vi "STED Control V1.vi"() -> ()   [LabVIEW 2014]
uses:
  FPGA-7842R-Reference.ctl
  Scan Parameters.ctl
  Manual Controls V2.ctl
  <vilib>/Utility/miscctls.llb/LVRectTypeDef.ctl
  <vilib>/Utility/miscctls.llb/LVPositionTypeDef.ctl
  Laser Controls.ctl
  Type Defs/Image Acquisition Parameters.ctl
  Detectors.ctl
panel:
  in  "Move XY Stage":bool
  in  "Autoscale Z":bool
  in  "Reset Zoom":bool
  in  "Zoom Out":bool
  in  "Zoom In":bool
  in  "Pan":bool
  in  "Remove Display":bool
  in  "Add Display":bool
  in  "Colormap 2":u16(ring) items=["Fire", "Gray", "Red", "Green", "Blue", "Cyan", "Magenta", "Yellow", "Red-White", "Green-White", "Blue-White", "Glow"]
  in  "Merge Tool":bool
  in  "Smooth Tool":bool
  out "Channel 6":sgl[][](graph)
  out "Channel 5":sgl[][](graph)
  out "Channel 4":sgl[][](graph)
  out "Channel 3":sgl[][](graph)
  out "Channel 2":sgl[][](graph)
  in  "Dual Screens":bool=TRUE
  in  "Detectors":T1
  in  "Laser Controls":T2 {"590 Power (V)" scale=0.0..3.0; "STED Power (V)" scale=0.0..5.0}
  in  "Save File Path":path
  in  "Capture":bool
  in  "show cursor":bool
  in  "Set Mode Offset":bool
  in  "Manual Controls":T3={"Galvo 1 Position (I16)"=-280, "Galvo 2 Position (I16)"=0, "X Axis Voltage (I16)"=16384, "Y Axis Voltage (I16)"=16384, "Z Axis Voltage (I16)"=16384, "Res Mirror Amp (I16)"=0, "Res Mirror Mute"=FALSE}
  in  "Unused Axis Voltage":i16=16300
  out "Channel 1":sgl[][](graph)
  in  "Image Acquisition Parameters":T4={"Scan Type"=enum."Sample Scanning", "Scan Mode"=enum."XY", "Fast Axis Frequency (Hz)"=100.0, "Image Format"=128, "Line Accumulations"=1, "Frames Per Capture"=1, "Frames Accumulations"=1, "Image Dimension (um)"=[], "Number of Z Steps"=1, "Z Steps Size (um)"=1.0, "Pixel Size (nm)"=[]} {"Z Steps Size (um)" min=0.0; "Number of Z Steps" min=1; "Frames Accumulations" min=1; "Frames Per Capture" min=1; "Line Accumulations" min=1; "Image Format" items=["64 x 64"=64, "128 x 128"=128, "256 x 256"=256, "512 x 512"=512, "1024 x 1024"=1024, "2048 x 2048"=2048]}
  in  "Live":bool
  in  "Exit":bool
  # "XY"
  # "Z"
  # "Length"
  # "Height"
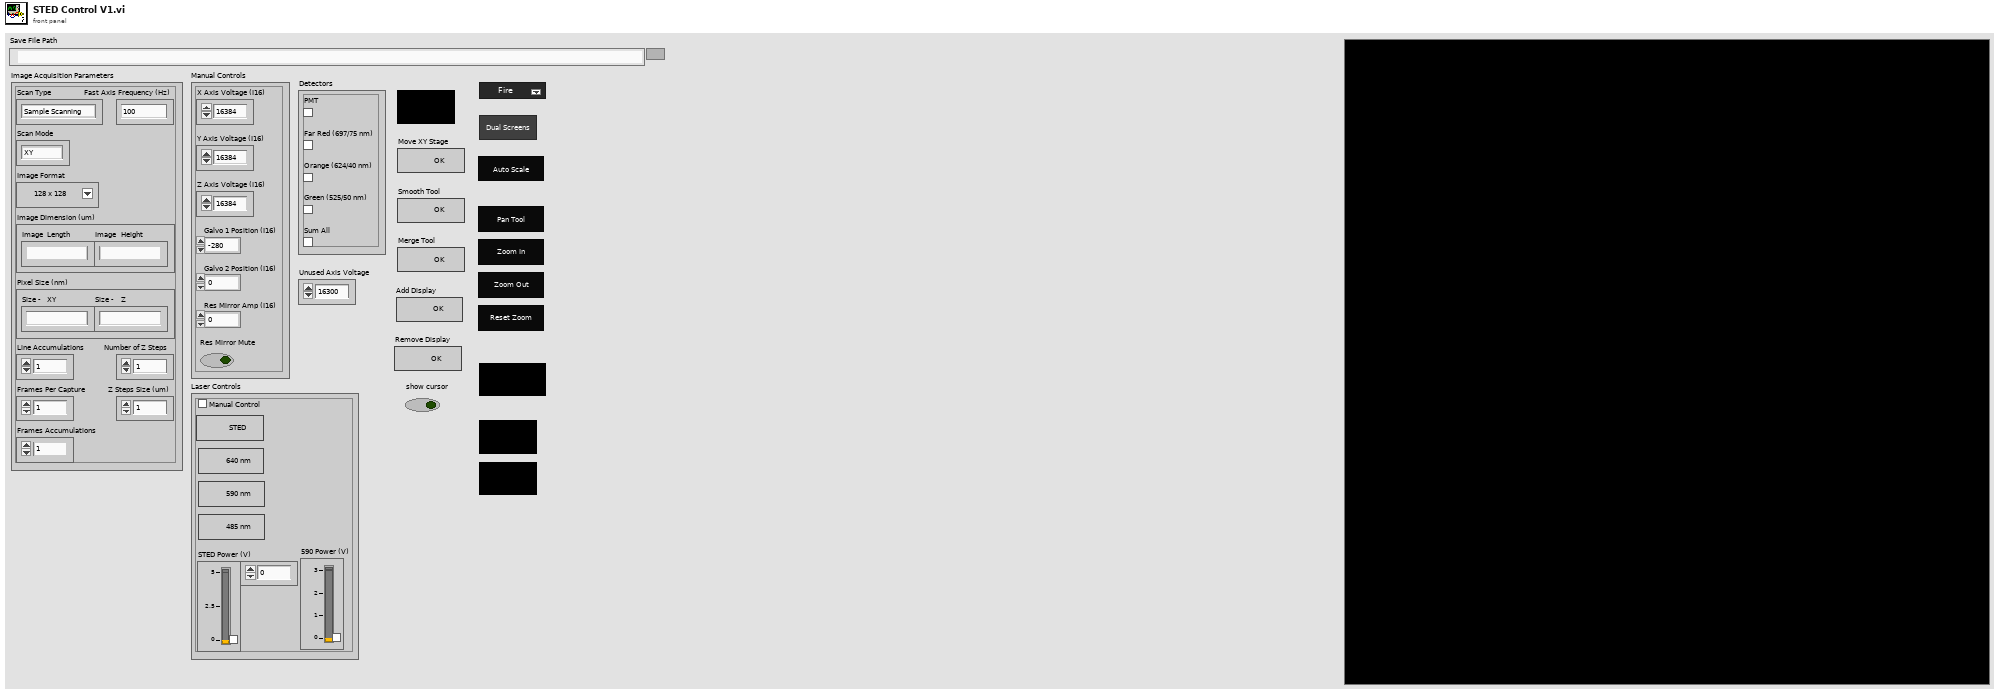
[diagram p1: front panel]
types:
  T1 = typedef "Detectors.ctl" = cluster{"PMT":bool, "Far Red (697/75 nm)":bool, "Orange (624/40 nm)":bool, "Green (525/50 nm)":bool, "Sum All":bool}
  T2 = typedef "Laser Controls.ctl" = cluster{"STED Power (V)":dbl, "590 Power (V)":dbl, "STED":bool, "640 nm":bool, "590 nm":bool, "485 nm":bool, "Manual Control":bool}
  T3 = typedef "Manual Controls V2.ctl" = cluster{"Galvo 1 Position (I16)":i16, "Galvo 2 Position (I16)":i16, "X Axis Voltage (I16)":i16, "Y Axis Voltage (I16)":i16, "Z Axis Voltage (I16)":i16, "Res Mirror Amp (I16)":i16, "Res Mirror Mute":bool}
  T4 = typedef "Image Acquisition Parameters.ctl" = cluster{"Scan Type":enum16{"Sample Scanning", "Beam Scanning"}, "Scan Mode":enum16{"XY", "XZ", "YZ", "XYZ"}, "Fast Axis Frequency (Hz)":dbl, "Image Format":u16, "Line Accumulations":u16, "Frames Per Capture":u16, "Frames Accumulations":u16, "Image Dimension (um)":dbl[], "Number of Z Steps":u8, "Z Steps Size (um)":dbl, "Pixel Size (nm)":dbl[]}
  T5 = typedef "Scan Parameters.ctl" = cluster{"Fast_Ax_Amp_V":dbl, "Fast_Ax_Off_V":dbl, "Slow_Ax_Amp_V":dbl, "Slow_Ax_Off_V ":dbl, "Slow_Ax_Max_V_VperS":dbl, "Slow_Ax1_Del25ns":i32, "Slow_Ax2_Del25ns":i32, "Stage_X_Off_V":dbl, "Stage_Y_Off_V":dbl, "Stage_Z_Off_V":dbl, "Galvo1_Off_V":dbl, "Galvo2_Off_V":dbl, "Last_Scan_Mode":enum16{"XY", "XZ", "YZ", "XYZ"}, "Current_Scan_Mode":enum16{"XY", "XZ", "YZ", "XYZ"}, "Fly_Back_Lines":u16, "Linear_Ramp_End":u32, "Z_Step_I16":i16, "Z_Start_I16":i16, "Laser_States _U32":u32, "590_Voltage_I16":i16, "775_AOM_Volt_I16":i16, "Blanking OFF":bool, "Unused_Axis_I16":i16}
  T6 = typedef "FPGA-7842R-Reference.ctl" = enum16{"Stage Control", "Laser Control", "Unused Axis I16", "Exit", "Set Res Mirror", "Set Galvo", "Default", "Close FPGA", "Stop Waveforms", "Start Waveforms", "Initialize"}
  T7 = typedef "LVPositionTypeDef.ctl" = cluster{"Left":i32, "Top":i32}
  T8 = typedef "LVRectTypeDef.ctl" = cluster{"Left":i16, "Top":i16, "Right":i16, "Bottom":i16}
  T9 = enum32{"Invalid", "Standard", "Closed", "Hidden", "Minimized", "Maximized"}
  T10 = typedef "LVRangeTypeDef.ctl" = cluster{"Minimum":dbl, "Maximum":dbl, "Increment":dbl, "Minor Increment":dbl, "Start":dbl}
  T11 = cluster{"Galvo 1 Position (I16)":bool, "Galvo 2 Position (I16)":bool, "X Axis Voltage (I16)":bool, "Y Axis Voltage (I16)":bool, "Z Axis Voltage (I16)":bool, "Res Mirror Amp (I16)":bool, "Res Mirror Mute":bool}
  T12 = typedef "LVAllMonitorsDisplayTypeDef.ctl" = cluster{"Bounds":cluster{"Left":i16, "Top":i16, "Right":i16, "Bottom":i16}, "Depth":i16}[]
  T13 = cluster{"Bounds":cluster{"Left":i16, "Top":i16, "Right":i16, "Bottom":i16}, "Depth":i16}
  T14 = typedef "Scanning Conversions.ctl" = cluster{"Stage X Axis (Volts/um)":dbl, "Stage Y Axis (Volts/um)":dbl, "Stage Z Axis (Volts/um)":dbl}
  T15 = typedef "IMAQ Image.ctl" = refnum<image>
  T16 = typedef "Waveform Data.ctl" = cluster{"Waveform Scan Parameters":cluster{"Scanning Mode":u8, "Fast Axis WF Length (Elements)":i32, "Fast Axis Sample Period (Ticks)":u32, "Slow Axis 1 WF Length (Elements)":i32, "Slow Axis 1 Sample Period (Ticks)":u32, "Slow Axis 1 Delay (25 ns) Steps":i32, "Slow Axis 2 WFLength (Elements)":i32, "Slow Axis 2 Sample Period (Ticks)":u32, "Slow Axis 2 Delay (25 ns) Steps":i32}, "Fast Axis Waveform":dbl[], "Slow Axis 1 Waveform":dbl[], "Slow Axis 2 Waveform":dbl[]}
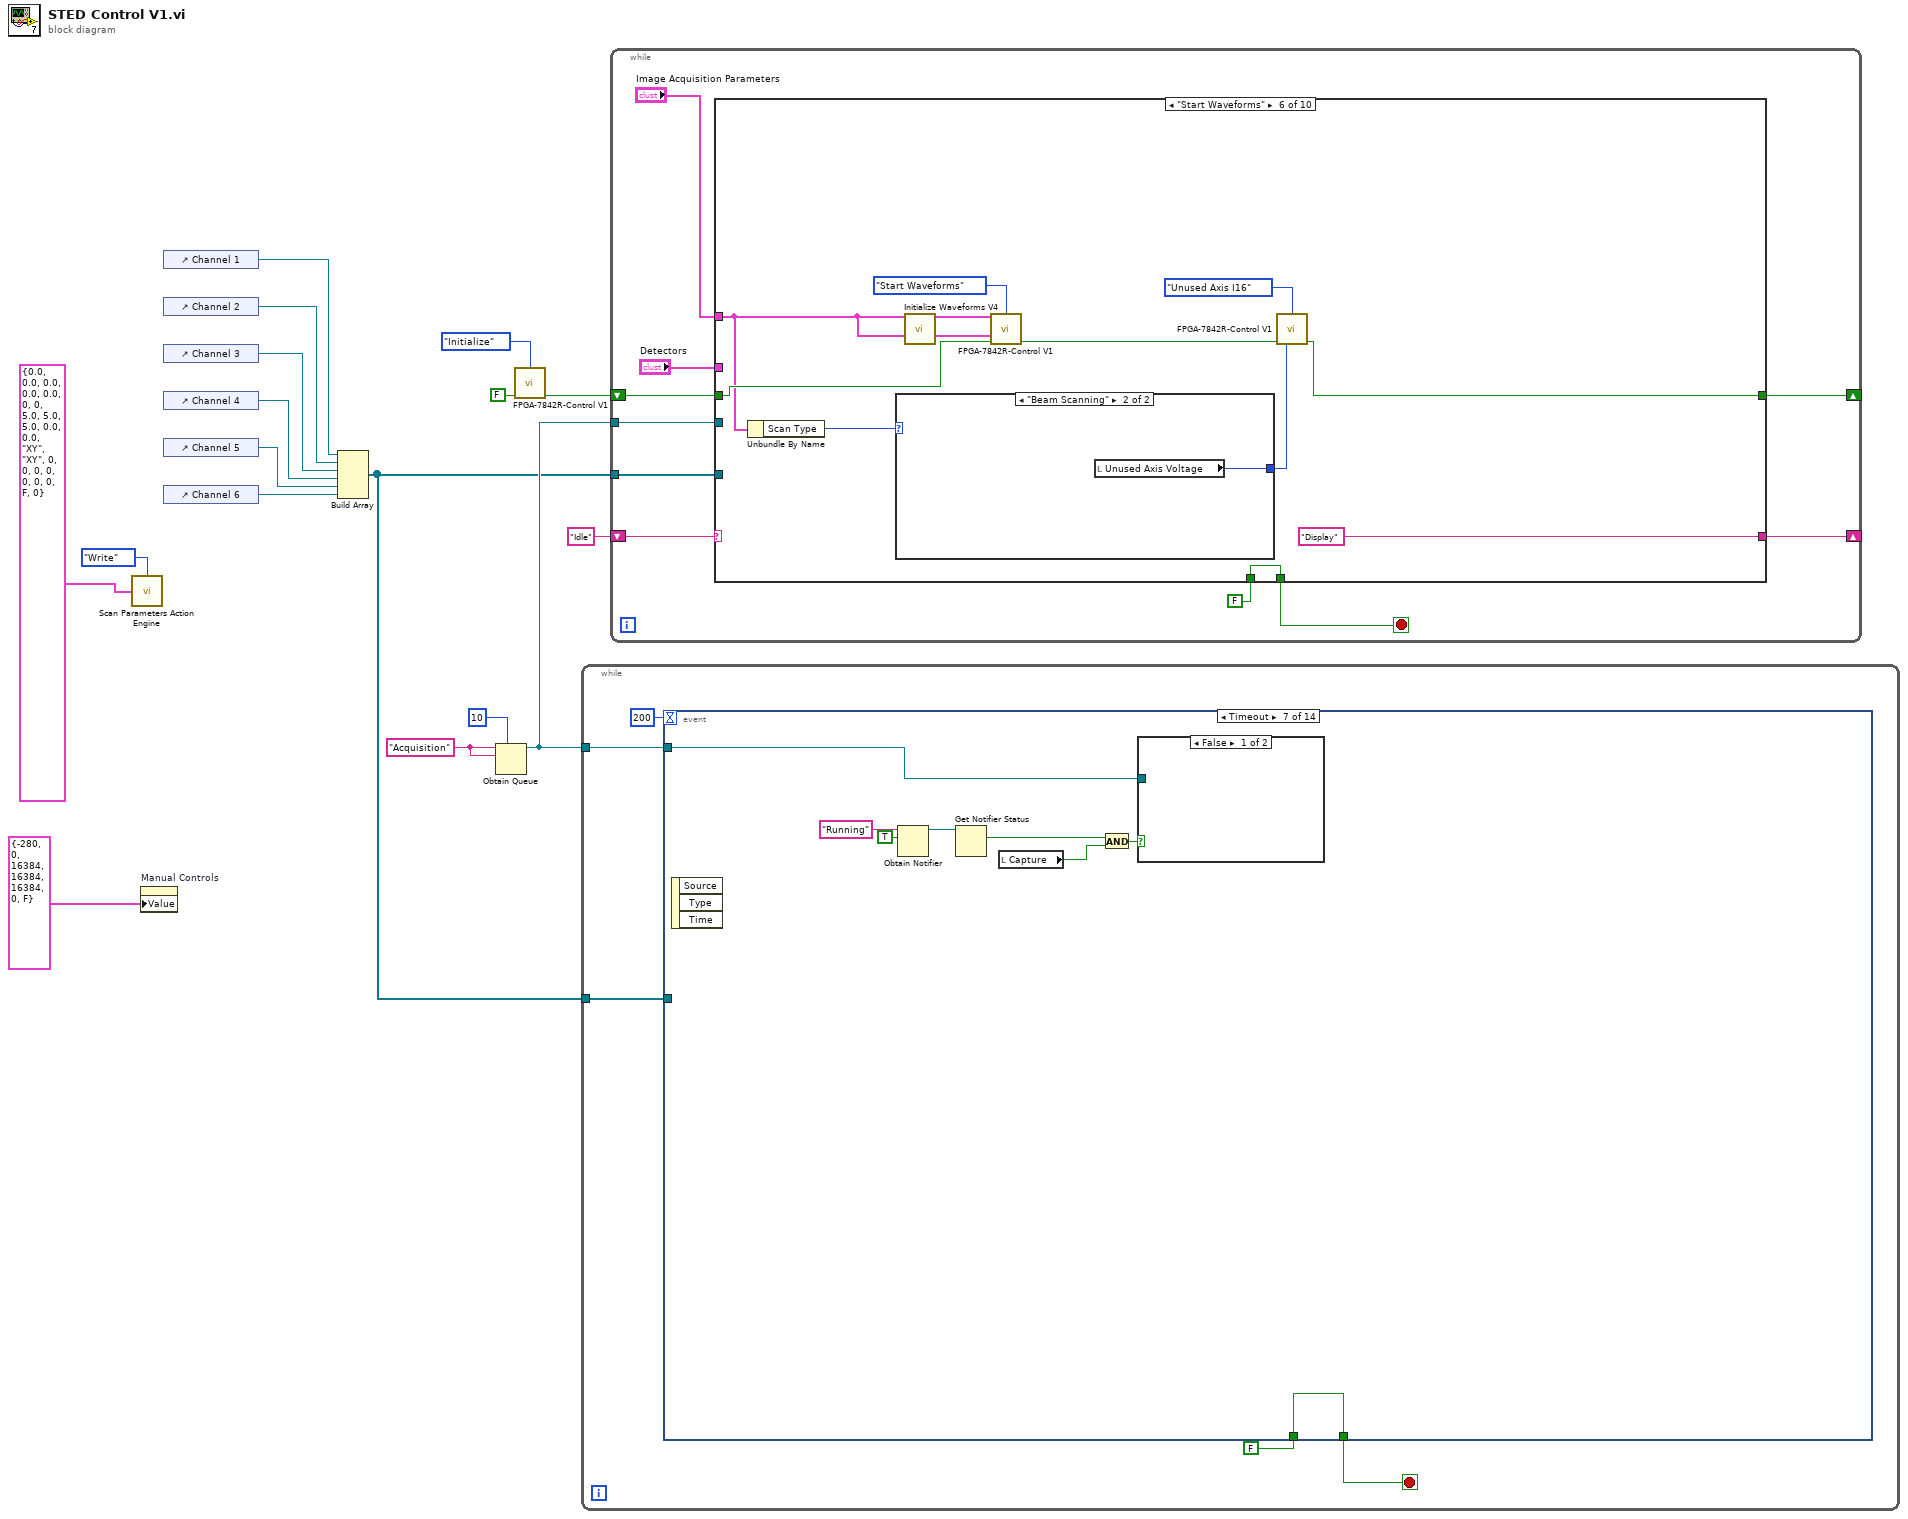
[diagram p0: block diagram]
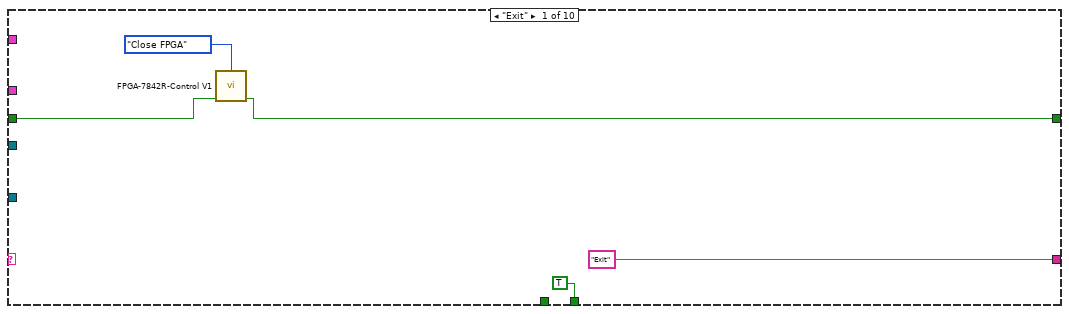
[diagram p2: hidden frame]
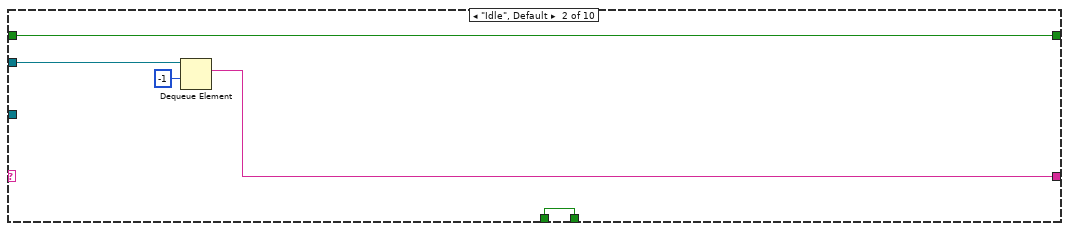
[diagram p3: hidden frame]
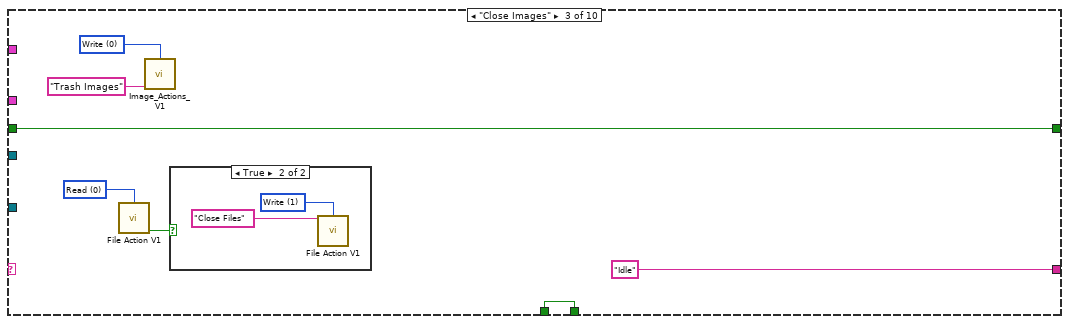
[diagram p4: hidden frame]
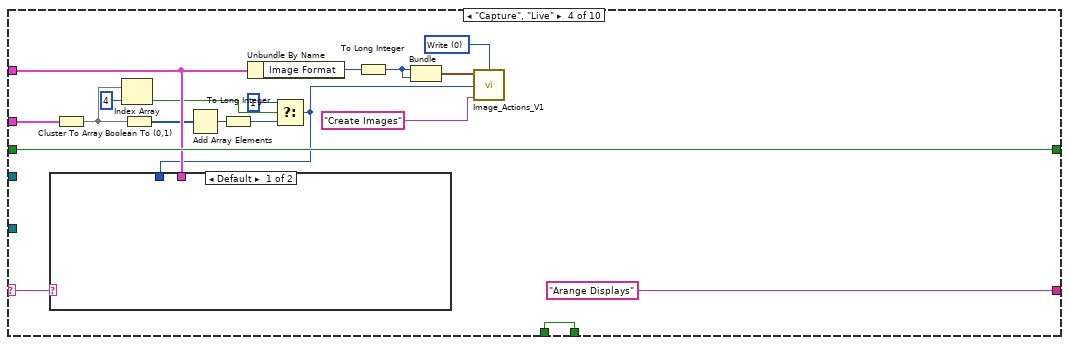
[diagram p6: hidden frame]
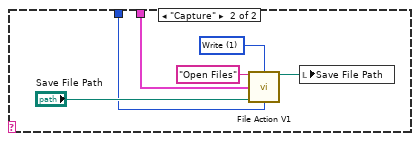
[diagram p7: hidden frame]
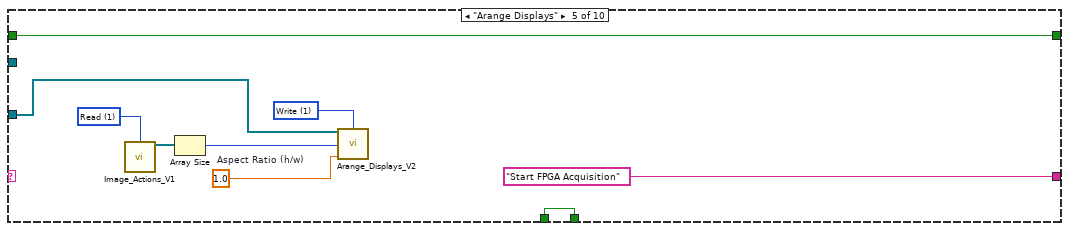
[diagram p8: hidden frame]
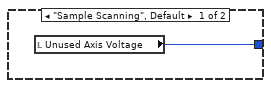
[diagram p9: hidden frame]
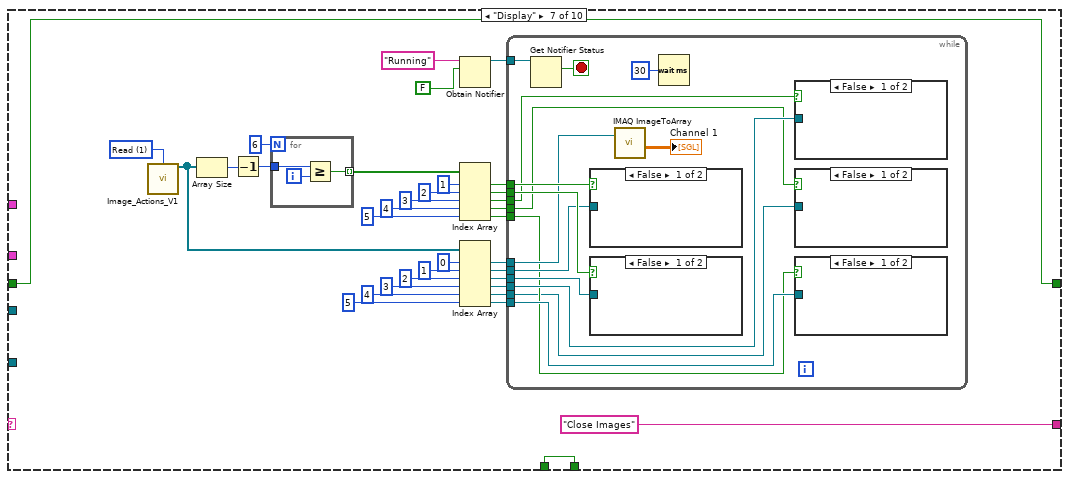
[diagram p10: hidden frame]
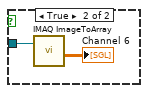
[diagram p11: hidden frame]
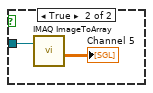
[diagram p12: hidden frame]
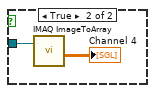
[diagram p13: hidden frame]
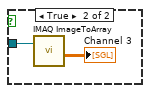
[diagram p14: hidden frame]
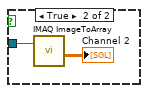
[diagram p15: hidden frame]
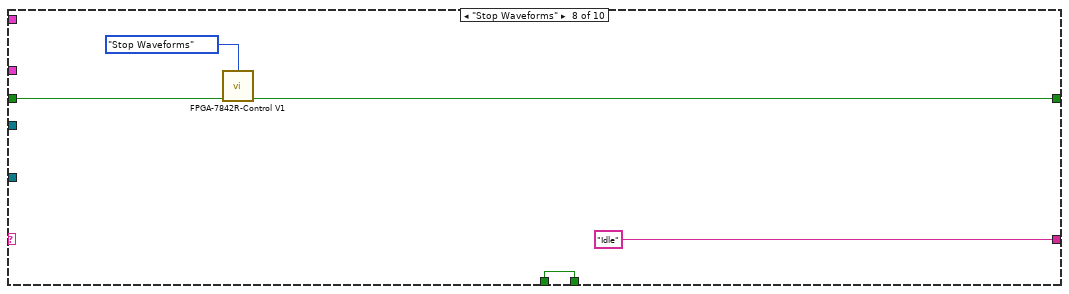
[diagram p16: hidden frame]
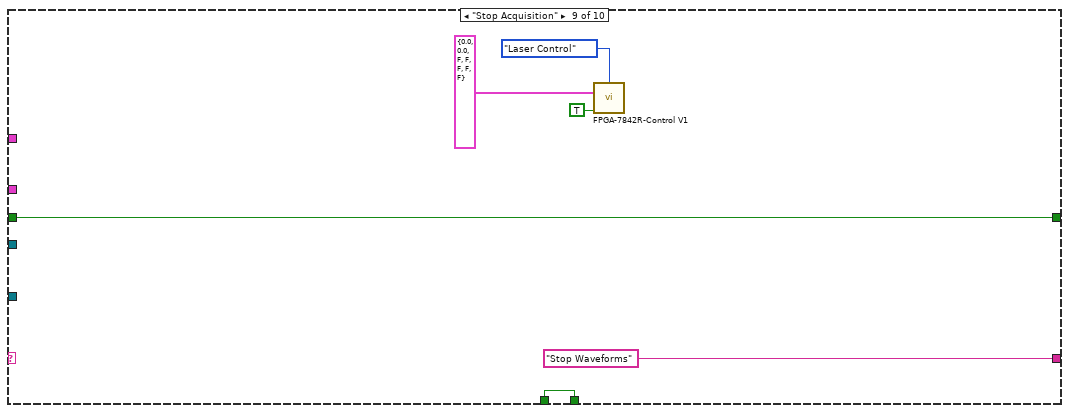
[diagram p17: hidden frame]
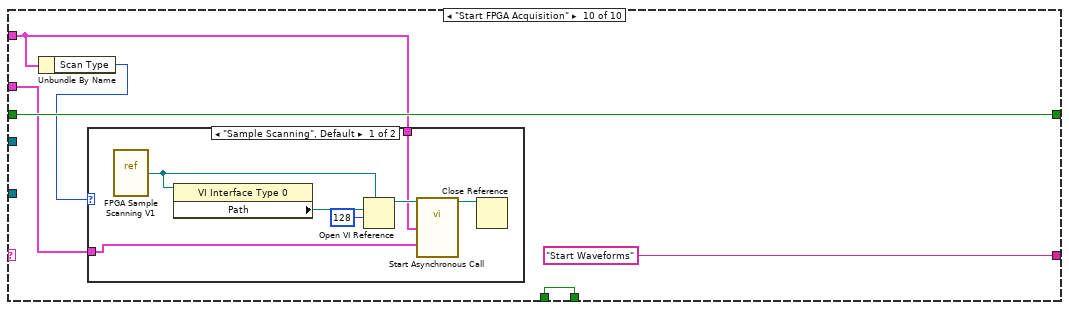
[diagram p18: hidden frame]
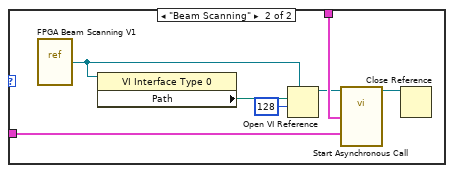
[diagram p19: hidden frame]
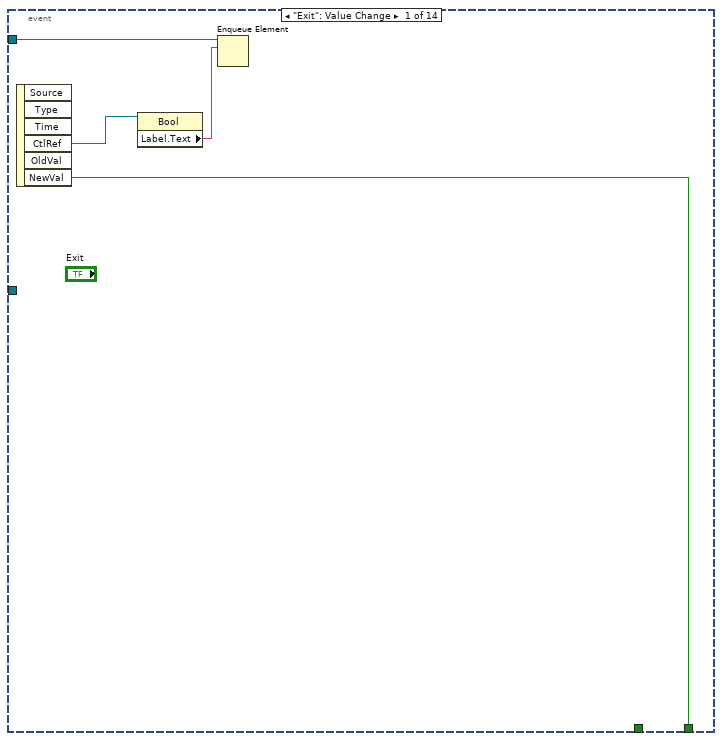
[diagram p20: hidden frame]
diagram:
  w16 = "Acquisition" ("name (unnamed)")
  n1 = call "Scan Parameters Action Engine.vi"("Action"=enum16{"Read", "Write"}."Write", "Scan Parameters IN"=T5 {"Fast_Ax_Amp_V"=0.0, "Fast_Ax_Off_V"=0.0, "Slow_Ax_Amp_V"=0.0, "Slow_Ax_Off_V "=0.0, "Slow_Ax_Max_V_VperS"=0.0, "Slow_Ax1_Del25ns"=0, "Slow_Ax2_Del25ns"=0, "Stage_X_Off_V"=5.0, "Stage_Y_Off_V"=5.0, "Stage_Z_Off_V"=5.0, "Galvo1_Off_V"=0.0, "Galvo2_Off_V"=0.0, "Last_Scan_Mode"=enum."XY", "Current_Scan_Mode"=enum."XY", "Fly_Back_Lines"=0, "Linear_Ramp_End"=0, "Z_Step_I16"=0, "Z_Start_I16"=0, "Laser_States _U32"=0, "590_Voltage_I16"=0, "775_AOM_Volt_I16"=0, "Blanking OFF"=FALSE, "Unused_Axis_I16"=0}) -> ()  [unwired: 13 in, 1 out]
  n2 = property on="Manual Controls" class="Clust (strict)"("Value"=T3 {"Galvo 1 Position (I16)"=-280, "Galvo 2 Position (I16)"=0, "X Axis Voltage (I16)"=16384, "Y Axis Voltage (I16)"=16384, "Z Axis Voltage (I16)"=16384, "Res Mirror Amp (I16)"=0, "Res Mirror Mute"=FALSE} ("Manual Controls")) -> ()  [unwired: 2 in, 2 out]
  n3 = control-ref of="Channel 1"() -> (w8:refnum<vi>)
  n4 = control-ref of="Channel 2"() -> (w7:refnum<vi>)
  n5 = control-ref of="Channel 3"() -> (w6:refnum<vi>)
  n6 = control-ref of="Channel 4"() -> (w5:refnum<vi>)
  n7 = control-ref of="Channel 5"() -> (w4:refnum<vi>)
  n8 = control-ref of="Channel 6"() -> (w3:refnum<vi>)
  n9 = Build Array(w8, w7, w6, w5, w4, w3) -> (w2:refnum<vi>[])
  n10 = Obtain Queue(max queue size (-1, unlimited)=10, name (unnamed)=w16, element data type=w16) -> (queue out=w14:refnum<queue>)  [unwired: 2 in, 2 out]
  n11 = call "FPGA-7842R-Control V1.vi"("Action"=FPGA-7842R-Reference."Initialize", "Initialize"=FALSE) -> ("Initalized"=w11:bool)  [unwired: 13 in]
  n12 = while {
    tunnel: w14 -> [w20]
    tunnel: w2 -> [w18]
    stop <- w22 stop-if-true
    n13 = event shown="[6] Timeout" {
      selector: _ -> [_ _ _ _ _ _ _ _ _ _ _ _ _ _]
      dyn-events: _ -> [_ _ _ _ _ _ _ _ _ _ _ _ _ _]
      timeout: 200 -> [_ _ _ _ _ _ _ _ _ _ _ _ _ _]
      tunnel: [w26 w38 w43 w81 w108 w173 w193 w208 w225 w252 w302 w431 w433 w645] -> w22
      tunnel: FALSE -> [_ w38 w43 w81 w108 w173 w193 w208 w225 w252 w302 w431 w433 w645]
      tunnel: w20 -> [w25 w37 _ _ _ _ w187 _ _ _ _ _ _ _]
      tunnel: w18 -> [_ _ w40 _ w103 w172 _ _ _ _ _ _ _ _]
      event "Exit": Value Change {
        n14 = event-data() -> ("CtlRef"=w24:refnum<vi>, "NewVal"=w26:bool)  [unwired: 1 in, 4 out]
        n15 = property class="Bool"(reference=w24) -> ("Label.Text"=w23:string)  [unwired: 1 in, 2 out]
        n16 = Enqueue Element(queue=w25, element=w23) -> ()  [unwired: 2 in, 3 out]
      }
      event "Live", "Capture": Value Change {
        n17 = event-data() -> ("CtlRef"=w36:refnum<vi>, "NewVal"=w28:bool)  [unwired: 1 in]
        n18 = property on="Channel 1" class="IntGraph (strict)"("Cursor.Visible"=FALSE) -> ()  [unwired: 2 in, 2 out]
        n19 = property class="Bool (strict)"(reference=w36) -> ("Label.Text"=w27:string)  [unwired: 1 in, 2 out]
        n20 = Obtain Notifier(name (unnamed)="Running", notification data type=TRUE) -> (notifier out=w33:refnum<notifier>)  [unwired: 2 in, 2 out]
        n21 = Not(x=w28) -> (.not. x?=w31:bool)
        n22 = Send Notification(notification=w31, notifier=w33) -> ()  [unwired: 1 in, 2 out]
        n23 = Select(t=w27, s=w28, f="Stop Acquisition") -> (s? t:f=w29:string)
        n24 = Enqueue Element(queue=w37, element=w29) -> ()  [unwired: 2 in, 3 out]
      }
      event "Smooth Tool", "Merge Tool", "Add Display", "Remove Display", "Autoscale Z", "Move XY Stage": Value Change {
        n25 = event-data() -> ("CtlRef"=w42:refnum<vi>)  [unwired: 1 in, 5 out]
        n26 = property class="Bool"(reference=w42) -> ("Label.Text"=w41:string)  [unwired: 1 in, 2 out]
        n27 = control-ref of="This VI"() -> (w39:refnum<vi>)
        n28 = case shown="\"Move XY Stage\"" w41 {
          tunnel: w40 -> [_ w45 w52 _ w62 w66 w72]
          tunnel: w39 -> [_ w44 _ _ _ _ w71]
          frame Default {
          }
          frame "Merge Tool" {
            n29 = vi-ref "MergeTool - Cambridge.vi"() -> (w49:refnum<vi>)
            n30 = property class="VI Interface Type 2"(reference=w49) -> ("Path"=w47:path)  [unwired: 1 in, 2 out]
            n31 = Open VI Reference(type specifier VI Refnum (for type only)=w49, vi path=w47, options=128) -> (vi reference=w48:refnum<vi>)  [unwired: 3 in, 1 out]
            n32 = call-by-ref "Start Asynchronous Call"(reference=w48, "VI Reference"=w44, "Display References"=w45) -> (reference out=w50:refnum<vi>)  [unwired: 11 in, 1 out]
            n33 = Close Reference(reference=w50) -> ()  [unwired: 1 in, 1 out]
          }
          frame "Add Display" {
            w55 = u16 1 items=["Read", "Write"] ("Action")
            w56 = u16 0 items=["Read", "Write"] ("Action")
            n34 = call "Arange_Displays_V2.vi"("Action"=w56) -> ("Number of Channels OUT"=w54:i32)  [unwired: 14 in]
            n35 = Increment(x=w54) -> (x+1=w53:i32)
            n36 = call "Arange_Displays_V2.vi"("Display References"=w52, "Action"=w55, "Number of Channels"=w53, "Aspect Ratio (h/w)"=1.0) -> ()  [unwired: 11 in, 1 out]
          }
          frame "Move XY Stage" {
            n37 = vi-ref "StageController_V2.vi"() -> (w60:refnum<vi>)
            n38 = property class="VI Interface Type 3"(reference=w60) -> ("Path"=w58:path)  [unwired: 1 in, 2 out]
            n39 = Open VI Reference(type specifier VI Refnum (for type only)=w60, vi path=w58, options=128) -> (vi reference=w59:refnum<vi>)  [unwired: 3 in, 1 out]
            n40 = call-by-ref "Start Asynchronous Call"(reference=w59) -> (reference out=w61:refnum<vi>)  [unwired: 13 in, 1 out]
            n41 = Close Reference(reference=w61) -> ()  [unwired: 1 in, 1 out]
          }
          frame "Autoscale Z" {
            n42 = for {
              tunnel: w62 -> [w63] mode=indexing
              n43 = property class="IntGraph (strict)"(reference=w63, "ZScale.ScaleFit"=u8 1 ("Z Scale.Scale Fit")) -> ()  [unwired: 1 in, 2 out]
            }
          }
          frame "Remove Display" {
            w69 = u16 1 items=["Read", "Write"] ("Action")
            w70 = u16 0 items=["Read", "Write"] ("Action")
            n44 = call "Arange_Displays_V2.vi"("Action"=w70) -> ("Number of Channels OUT"=w68:i32)  [unwired: 14 in]
            n45 = Decrement(x=w68) -> (x-1=w67:i32)
            n46 = call "Arange_Displays_V2.vi"("Display References"=w66, "Action"=w69, "Number of Channels"=w67, "Aspect Ratio (h/w)"=1.0) -> ()  [unwired: 11 in, 1 out]
          }
          frame "Smooth Tool" {
            n47 = vi-ref "SmoothTool.vi"() -> (w74:refnum<vi>)
            n48 = property class="VI Interface Type 3"(reference=w74) -> ("Path"=w76:path)  [unwired: 1 in, 2 out]
            n49 = Open VI Reference(type specifier VI Refnum (for type only)=w74, vi path=w76, options=128) -> (vi reference=w75:refnum<vi>)  [unwired: 3 in, 1 out]
            n50 = call-by-ref "Start Asynchronous Call"(reference=w75, "VI Reference"=w71, "Display References"=w72) -> (reference out=w73:refnum<vi>)  [unwired: 2 in, 1 out]
            n51 = Close Reference(reference=w73) -> ()  [unwired: 1 in, 1 out]
          }
        }
      }
      event "Pan", "Zoom In", "Zoom Out", "Reset Zoom": Value Change {
        n52 = event-data() -> ("CtlRef"=w79:refnum<vi>, "NewVal"=w78:bool)  [unwired: 1 in]
        n53 = case shown="True" w78 {
          tunnel: w79 -> [_ w89]
          tunnel: [0 ("Palette:Active Tool") w88] -> w80
          frame False {
          }
          frame True {
            n54 = property class="Bool (strict)"(reference=w89) -> ("Label.Text"=w83:string)  [unwired: 1 in, 2 out]
            n55 = Build Array("Pan", "Zoom In", "Zoom Out") -> (w84:string[])
            n56 = case shown="\"Pan\"" w83 {
              tunnel: [6 ("Palette:Active Tool") 7 ("Palette:Active Tool") 5 ("Palette:Active Tool") 1 ("Palette:Active Tool")] -> w88
              frame "Zoom In" {
              }
              frame "Zoom Out" {
              }
              frame "Reset Zoom", Default {
              }
              frame "Pan" {
              }
            }
            n57 = for {
              tunnel: w84 -> [w90] mode=indexing
              tunnel: w83 -> [w94]
              n58 = Equal?(x=w94, y=w90) -> (x = y?=w91:bool)
              n59 = control-ref of="This VI"() -> (w92:refnum<vi>)
              n60 = To Variant(anything=w91) -> (Variant=w93:variant)
              n61 = invoke class="VI" method="Ctrl Val.Set"(reference=w92, "Control Name"=w90, "Value"=w93) -> ()  [unwired: 2 in, 5 out]
            }
          }
        }
        n62 = property on="Channel 1" class="IntGraph (strict)"("ActPaletteTool"=w80) -> ()  [unwired: 2 in, 2 out]
        n63 = property on="Channel 2" class="IntGraph (strict)"("ActPaletteTool"=w80) -> ()  [unwired: 2 in, 2 out]
        n64 = property on="Channel 3" class="IntGraph (strict)"("ActPaletteTool"=w80) -> ()  [unwired: 2 in, 2 out]
        n65 = property on="Channel 4" class="IntGraph (strict)"("ActPaletteTool"=w80) -> ()  [unwired: 2 in, 2 out]
        n66 = property on="Channel 5" class="IntGraph (strict)"("ActPaletteTool"=w80) -> ()  [unwired: 2 in, 2 out]
        n67 = property on="Channel 6" class="IntGraph (strict)"("ActPaletteTool"=w80) -> ()  [unwired: 2 in, 2 out]
      }
      event "Channel 1", "Channel 2", "Channel 3", "Channel 4", "Channel 5", "Channel 6": Mouse Down {
        n68 = event-data() -> ("CtlRef"=w104:refnum<vi>, "Mods.Double Click"=w107:bool, "PlatMods.Shift"=w106:bool, "PlatMods.Ctrl"=w105:bool)  [unwired: 1 in]
        n69 = Build Array(w107, w106, w105) -> (w100:bool[])
        n70 = property class="IntGraph (strict)"(reference=w104) -> (reference out=w102:refnum<vi>, "Label.Text"=w99:string)  [unwired: 1 in, 1 out]
        n71 = Boolean Array To Number(Boolean array=w100) -> (number=w101:u32)
        n72 = case shown="0" w101 {
          tunnel: w99 -> [w110 _ _ _ _]
          tunnel: w102 -> [_ w125 w160 w171 _]
          tunnel: w103 -> [w109 _ _ _ _]
          frame 0 {
            n73 = for {
              tunnel: w110 -> [w114]
              tunnel: w109 -> [w113] mode=indexing
              # "Single Click - Show Z Scale"
              n74 = property class="IntGraph (strict)"(reference=w113) -> (reference out=w111:refnum<vi>, "Label.Text"=w112:string)  [unwired: 1 in, 1 out]
              n75 = Equal?(x=w112, y=w114) -> (x = y?=w116:bool)
              n76 = Select(t=T7 {"Left"=2000, "Top"=17} ("Z Scale.Position"), s=w116, f=T7 {"Left"=0, "Top"=0} ("Z Scale.Position")) -> (s? t:f=w115:T7)
              n77 = property class="IntGraph (strict)"(reference=w111, "ZScale.Visible"=w116, "ZScale.Position"=w115) -> ()  [unwired: 1 in, 2 out]
            }
          }
          frame 2 {
            # "Shift Click - Apply color map."
            n78 = property class="IntGraph (strict)"(reference=w125) -> (reference out=w119:refnum<vi>, "ZScale.Maximum"=w120:dbl)  [unwired: 1 in, 1 out]
            n79 = case shown="0, Default" "Colormap 2" {
              tunnel: [cluster{dbl, u32}[] [{0.0, 0}, {85.0, 16711680}, {108.0, 16729344}, {127.0, 16744192}, {132.0, 16747520}, {140.0, 16753920}, {157.0, 16766720}, {170.0, 16776960}, {245.0, 16777184}, {250.0, 16777200}, {255.0, 16777215}] ("Z Scale.Marker Values[]") cluster{dbl, u32}[] [{0.0, 0}, {255.0, 16777215}] ("Z Scale.Marker Values[]") cluster{dbl, u32}[] [{0.0, 0}, {255.0, 16711680}] ("Z Scale.Marker Values[]") cluster{dbl, u32}[] [{0.0, 0}, {255.0, 65280}] ("Z Scale.Marker Values[]") cluster{dbl, u32}[] [{0.0, 0}, {255.0, 255}] ("Z Scale.Marker Values[]") cluster{dbl, u32}[] [{0.0, 0}, {255.0, 65535}] ("Z Scale.Marker Values[]") cluster{dbl, u32}[] [{0.0, 0}, {255.0, 16711935}] ("Z Scale.Marker Values[]") cluster{dbl, u32}[] [{0.0, 0}, {255.0, 16776960}] ("Z Scale.Marker Values[]") cluster{dbl, u32}[] [{0.0, 0}, {170.0, 16711680}, {245.0, 16777184}, {250.0, 16777200}, {255.0, 16448250}] ("Z Scale.Marker Values[]") cluster{dbl, u32}[] [{0.0, 0}, {170.0, 65280}, {245.0, 16777184}, {250.0, 16777200}, {255.0, 16448250}] ("Z Scale.Marker Values[]") cluster{dbl, u32}[] [{0.0, 0}, {170.0, 255}, {245.0, 16777184}, {250.0, 16777200}, {255.0, 16448250}] ("Z Scale.Marker Values[]") cluster{dbl, u32}[] [{0.0, 0}, {1.0, 131072}, {2.0, 196608}, {3.0, 327680}, {4.0, 458752}, {5.0, 589824}, {6.0, 720896}, {7.0, 851971}, {8.0, 983043}, {9.0, 1114115}, {10.0, 1245187}, {11.0, 1376259}, {12.0, 1507331}, {13.0, 1638403}, {14.0, 1769475}, {15.0, 1769479}, {16.0, 2031623}, {17.0, 2162695}, {18.0, 2293767}, {19.0, 2424839}, {20.0, 2555911}, {21.0, 2686983}, {22.0, 2818055}, {23.0, 2949127}, {24.0, 3080203}, {25.0, 3211275}, {26.0, 3342347}, {27.0, 3473419}, {28.0, 3604491}, {29.0, 3735563}, {30.0, 3866635}, {31.0, 3867403}, {32.0, 4129547}, {33.0, 4260619}, {34.0, 4391691}, {35.0, 4522763}, {36.0, 4653839}, {37.0, 4784911}, {38.0, 4915983}, {39.0, 5178127}, {40.0, 5309199}, {41.0, 5440271}, {42.0, 5571343}, {43.0, 5702415}, {44.0, 5703439}, {45.0, 5965583}, {46.0, 6096655}, {47.0, 6227727}, {48.0, 6358799}, {49.0, 6489871}, {50.0, 6620943}, {51.0, 6752015}, {52.0, 6883087}, {53.0, 7015183}, {54.0, 7146255}, {55.0, 7277327}, {56.0, 7408399}, {57.0, 7539471}, {58.0, 7670543}, {59.0, 7801615}, {60.0, 8063759}, {61.0, 8194831}, {62.0, 8326927}, {63.0, 8457999}, {64.0, 8589075}, {65.0, 8720147}, {66.0, 8851219}, {67.0, 8982291}, {68.0, 9113363}, {69.0, 9114387}, {70.0, 9376531}, {71.0, 9507603}, {72.0, 9638675}, {73.0, 9769747}, {74.0, 9901843}, {75.0, 10032915}, {76.0, 10163987}, {77.0, 10229523}, {78.0, 10295059}, {79.0, 10427155}, {80.0, 10558227}, {81.0, 10689299}, {82.0, 10820371}, {83.0, 10886931}, {84.0, 10952467}, {85.0, 11083539}, {86.0, 11214611}, {87.0, 11215635}, {88.0, 11477779}, {89.0, 11543315}, {90.0, 11608851}, {91.0, 11740947}, {92.0, 11806483}, {93.0, 11872019}, {94.0, 12004115}, {95.0, 12135187}, {96.0, 12266259}, {97.0, 12267283}, {98.0, 12398355}, {99.0, 12529427}, {100.0, 12530451}, {101.0, 12595987}, {102.0, 12530451}, {103.0, 12793619}, {104.0, 12794131}, {105.0, 12794643}, {106.0, 13056787}, {107.0, 13057299}, {108.0, 13057811}, {109.0, 13188883}, {110.0, 13320979}, {111.0, 13386515}, {112.0, 13452563}, {113.0, 13584147}, {114.0, 13584659}, {115.0, 13585171}, {116.0, 13585683}, {117.0, 13717267}, {118.0, 13848339}, {119.0, 13849363}, {120.0, 13849875}, {121.0, 13850387}, {122.0, 13981459}, {123.0, 14113555}, {124.0, 14114067}, {125.0, 14114579}, {126.0, 14115091}, {127.0, 14246675}, {128.0, 14377747}, {129.0, 14378771}, {130.0, 14379283}, {131.0, 14379539}, {132.0, 14379795}, {133.0, 14380819}, {134.0, 14511891}, {135.0, 14643987}, {136.0, 14644503}, {137.0, 14645015}, {138.0, 14645527}, {139.0, 14646039}, {140.0, 14646551}, {141.0, 14778135}, {142.0, 14909207}, {143.0, 14910231}, {144.0, 14910747}, {145.0, 14911259}, {146.0, 14911771}, {147.0, 14912283}, {148.0, 14912797}, {149.0, 15044383}, {150.0, 15175455}, {151.0, 15175967}, {152.0, 15176479}, {153.0, 15176991}, {154.0, 15177507}, {155.0, 15178019}, {156.0, 15178531}, {157.0, 15310115}, {158.0, 15441701}, {159.0, 15441959}, {160.0, 15442215}, {161.0, 15442727}, {162.0, 15443243}, {163.0, 15443755}, {164.0, 15444269}, {165.0, 15444783}, {166.0, 15444783}, {167.0, 15576367}, {168.0, 15707953}, {169.0, 15708467}, {170.0, 15708979}, {171.0, 15708981}, {172.0, 15708983}, {173.0, 15710011}, {174.0, 15710523}, {175.0, 15711037}, {176.0, 15711039}, {177.0, 15711553}, {178.0, 15843139}, {179.0, 15974213}, {180.0, 15974215}, {181.0, 15974217}, {182.0, 15974219}, {183.0, 15975755}, {184.0, 15976271}, {185.0, 15976785}, {186.0, 15977299}, {187.0, 15977301}, {188.0, 15977815}, {189.0, 15978327}, {190.0, 15978331}, {191.0, 16109917}, {192.0, 16241503}, {193.0, 16241505}, {194.0, 16242019}, {195.0, 16242535}, {196.0, 16242537}, {197.0, 16242539}, {198.0, 16243563}, {199.0, 16243567}, {200.0, 16244081}, {201.0, 16244595}, {202.0, 16244599}, {203.0, 16244601}, {204.0, 16244603}, {205.0, 16245627}, {206.0, 16245631}, {207.0, 16245633}, {208.0, 16246147}, {209.0, 16246663}, {210.0, 16377735}, {211.0, 16508811}, {212.0, 16508815}, {213.0, 16509839}, {214.0, 16509843}, {215.0, 16509845}, {216.0, 16509847}, {217.0, 16510361}, {218.0, 16510875}, {219.0, 16510879}, {220.0, 16510881}, {221.0, 16510883}, {222.0, 16511399}, {223.0, 16511911}, {224.0, 16511915}, {225.0, 16511917}, {226.0, 16511919}, {227.0, 16511923}, {228.0, 16512437}, {229.0, 16512951}, {230.0, 16512955}, {231.0, 16512957}, {232.0, 16512959}, {233.0, 16512961}, {234.0, 16512963}, {235.0, 16512967}, {236.0, 16513481}, {237.0, 16513995}, {238.0, 16513999}, {239.0, 16514001}, {240.0, 16514003}, {241.0, 16514005}, {242.0, 16514007}, {243.0, 16514011}, {244.0, 16514013}, {245.0, 16514015}, {246.0, 16514019}, {247.0, 16514021}, {248.0, 16514023}, {249.0, 16514027}, {250.0, 16514029}, {251.0, 16514031}, {252.0, 16514035}, {253.0, 16514037}, {254.0, 16514039}, {255.0, 16514043}] ("Z Scale.Marker Values[]")] -> w123
              tunnel: w120 -> [w126 w128 w130 w132 w134 w136 w138 w140 w142 w144 w146 w149]
              tunnel: [w126 w128 w130 w132 w134 w136 w138 w140 w142 w144 w146 w149] -> w124
              frame 0, Default {
                # "Fire"
              }
              frame 1 {
                # "Grayscale"
              }
              frame 2 {
                # "Red"
              }
              frame 3 {
                # "Green"
              }
              frame 4 {
                # "Blue"
              }
              frame 5 {
                # "Cyan"
              }
              frame 6 {
                # "Magenta"
              }
              frame 7 {
                # "Yellow"
              }
              frame 8 {
                # "Red-White"
              }
              frame 9 {
                # "Green-White"
              }
              frame 10 {
                # "Blue-White"
              }
              frame 11 {
              }
            }
            n80 = property class="IntGraph (strict)"(reference=w119, "ZScale.MarkerVals[]"=w123, "ZScale.High Color"=u32 255, "ZScale.Maximum"=w124) -> ()  [unwired: 1 in, 2 out]
          }
          frame 6 {
            w159 = u16 1 items=["Get Image", "Load and Read File"] ("Action")
            # "Shift Control Click - Open Image"
            n81 = call "OpenDBL.vi"("Action"=w159) -> ("Image"=w158:sgl[], "Dimensions (Z, Y, X, t)"=w157:i32[])  [unwired: 12 in, 1 out]
            n82 = Index Array(array=w157, index #1=1 ("index"), index #2=2 ("index")) -> (element #1=w154:i32, element #2=w152:i32)
            n83 = Reverse 1D Array(array=w158) -> (reversed array=w151:sgl[])
            n84 = Reshape Array(w151, w154, w152) -> (w153:sgl[][])
            n85 = Transpose 2D Array(2D array=w153) -> (transposed array=w150:sgl[][])
            n86 = property class="IntGraph (strict)"(reference=w160, "Value"=w150) -> ()  [unwired: 1 in, 2 out]
          }
          frame 4 {
            # "Control Click - Open for feature fitting"
            n87 = property class="IntGraph (strict)"(reference=w171) -> ("Value"=w165:sgl[][])  [unwired: 1 in, 2 out]
            n88 = local read "Image Acquisition Parameters"() -> (w164:T4)
            n89 = vi-ref "QuickProfile_V3.vi"() -> (w170:refnum<vi>)
            n90 = property class="VI Interface Type 5"(reference=w170) -> ("Path"=w167:path)  [unwired: 1 in, 2 out]
            n91 = Unbundle By Name(w164) -> ("Pixel Size (nm)"=w163:dbl[])
            n92 = Index Array(array=w163, index=0) -> (element=w161:dbl)
            n93 = Open VI Reference(type specifier VI Refnum (for type only)=w170, vi path=w167, options=128) -> (vi reference=w169:refnum<vi>)  [unwired: 3 in, 1 out]
            n94 = call-by-ref "Start Asynchronous Call"(reference=w169, "Image IN"=w165, "Pixel Size (nm)"=w161) -> (reference out=w166:refnum<vi>)  [unwired: 15 in, 1 out]
            n95 = Close Reference(reference=w166) -> ()  [unwired: 1 in, 1 out]
          }
          frame 10, Default {
            # "No match case"
          }
        }
      }
      event "Channel 1", "Channel 2", "Channel 3", "Channel 4", "Channel 5", "Channel 6": Mouse Up {
        n96 = event-data() -> ("CtlRef"=w174:refnum<vi>)  [unwired: 1 in]
        n97 = property class="IntGraph (strict)"(reference=w174) -> (reference out=w175:refnum<vi>, "ActPaletteTool"=w178:i32)  [unwired: 1 in, 1 out]
        n98 = Not Equal?(x=w178, y=0) -> (x != y?=w176:bool)
        n99 = case shown="True" w176 {
          tunnel: w175 -> [_ w182]
          tunnel: w172 -> [_ w179]
          frame False {
          }
          frame True {
            n100 = property class="IntGraph (strict)"(reference=w182) -> ("XScale.Range"=w181:T10, "YScale.Range"=w180:T10)  [unwired: 1 in, 2 out]
            n101 = for {
              tunnel: w181 -> [w184]
              tunnel: w180 -> [w185]
              tunnel: w179 -> [w183] mode=indexing
              n102 = property class="IntGraph (strict)"(reference=w183, "XScale.Range"=w184, "YScale.Range"=w185) -> ()  [unwired: 1 in, 2 out]
            }
          }
        }
      }
      event Timeout {
        n103 = event-data() -> ()  [unwired: 1 in, 3 out]
        n104 = Obtain Notifier(name (unnamed)="Running", notification data type=TRUE) -> (notifier out=w191:refnum<notifier>)  [unwired: 2 in, 2 out]
        n105 = Get Notifier Status(notifier=w191) -> (current notification=w189:bool)  [unwired: 1 in, 4 out]
        n106 = local read "Capture"() -> (w188:bool)
        n107 = And(x=w189, y=w188) -> (x .and. y?=w186:bool)
        n108 = case shown="False" w186 {
          tunnel: w187 -> [_ w195]
          frame False {
          }
          frame True {
            n109 = local write "Capture"(FALSE ("Capture")) -> ()
            n110 = Enqueue Element(queue=w195, element="Stop Acquisition" ("f")) -> ()  [unwired: 2 in, 3 out]
          }
        }
      }
      event Value Change {
        n111 = event-data() -> ("CtlRef"=w202:refnum<vi>, "OldVal"=w203:T3, "NewVal"=w199:T3)  [unwired: 1 in, 3 out]
        n112 = Not Equal?(x=w203, y=w199) -> (x != y?=w204:T11)
        n113 = property class="Clust (strict)"(reference=w202) -> ("Controls[]"=w205:refnum<vi>[])  [unwired: 1 in, 2 out]
        n114 = Cluster To Array(cluster=w204) -> (array=w206:bool[])
        n115 = for {
          tunnel: w205 -> [w219] mode=indexing
          tunnel: w206 -> [w220] mode=indexing
          tunnel: [w219] -> w207
          stop <- w220 stop-if-true
        }
        n116 = property class="Ctl"(reference=w207) -> ("Label.Text"=w201:string)  [unwired: 1 in, 2 out]
        n117 = case shown="\"Z Axis Voltage (I16)\"" w201 {
          tunnel: [FPGA-7842R-Reference."Exit" ("Action") FPGA-7842R-Reference."Stage Control" ("Action") FPGA-7842R-Reference."Stage Control" ("Action") FPGA-7842R-Reference."Stage Control" ("Action") FPGA-7842R-Reference."Set Galvo" ("Action") FPGA-7842R-Reference."Set Galvo" ("Action") FPGA-7842R-Reference."Set Res Mirror" ("Action") FPGA-7842R-Reference."Set Res Mirror" ("Action") FPGA-7842R-Reference."Stage Control" ("Action") FPGA-7842R-Reference."Stage Control" ("Action")] -> w200
          frame Default {
          }
          frame "X Axis Voltage (I16)" {
          }
          frame "Y Axis Voltage (I16)" {
          }
          frame "Z Axis Voltage (I16)" {
          }
          frame "Galvo 1 Position (I16)" {
          }
          frame "Galvo 2 Position (I16)" {
          }
          frame "Res Mirror Amp (I16)" {
          }
          frame "Res Mirror Mute" {
          }
          frame "AOM (Pin 51 AO4)" {
          }
          frame "Beam Blanking" {
          }
        }
        n118 = call "FPGA-7842R-Control V1.vi"("Action"=w200, "Manual Controls"="Manual Controls", "Initialize"=TRUE) -> ()  [unwired: 12 in, 1 out]
      }
      event Value Change {
        w238 = FALSE ("element")
        n119 = event-data() -> ()  [unwired: 1 in, 6 out]
        n120 = Unbundle By Name("Laser Controls") -> ("STED"=w244:bool, "640 nm"=w241:bool, "590 nm"=w242:bool, "485 nm"=w243:bool, "590 Power (V)"=w235:dbl, "STED Power (V)"=w234:dbl, "Manual Control"=w222:bool)
        n121 = Build Array(w244, w241, w242, w243, w238, w238, w238, w238) -> (w240:bool[])
        n122 = local read "Live"() -> (w223:bool)
        n123 = Boolean Array To Number(Boolean array=w240) -> (number=w239:u32)
        n124 = To Unsigned Byte Integer(number=w239) -> (unsigned 8bit integer=w237:u8)
        n125 = Or(x=w223, y=w222) -> (x .or. y?=w221:bool)
        n126 = call "U8_To_U32.vi"("U8 IN"=w237) -> ("U32 OUT"=w236:u32)  [unwired: 13 in, 1 out]
        n127 = case shown="True" w221 {
          tunnel: "Laser Controls" -> [_ w250]
          frame False {
          }
          frame True {
            n128 = call "FPGA-7842R-Control V1.vi"("Action"=FPGA-7842R-Reference."Laser Control", "Laser Controls"=w250, "Initialize"=TRUE) -> ()  [unwired: 12 in, 1 out]
          }
        }
        n129 = In Range and Coerce(upper limit=3.0, x=w235, lower limit=0.0) -> (coerced(x)=w229:dbl)  [unwired: 1 out]
        n130 = In Range and Coerce(upper limit=5.0, x=w234, lower limit=0.0) -> (coerced(x)=w228:dbl)  [unwired: 1 out]
        n131 = call "Volts to I16.vi"("Voltage (V)"=w229) -> ("I16"=w227:i16)  [unwired: 13 in, 1 out]
        n132 = call "Volts to I16.vi"("Voltage (V)"=w228) -> ("I16"=w226:i16)  [unwired: 13 in, 1 out]
        n133 = call "Scan Parameters Action Engine.vi"("Action"=enum16{"Read", "Write"}."Read") -> ("Scan Parameters OUT"=w247:T5)  [unwired: 14 in]
        n134 = Bundle By Name(cluster=w247, "Laser_States _U32"=w236, "590_Voltage_I16"=w227, "775_AOM_Volt_I16"=w226) -> (w245:T5)
        n135 = call "Scan Parameters Action Engine.vi"("Action"=enum16{"Read", "Write"}."Write", "Scan Parameters IN"=w245) -> ()  [unwired: 13 in, 1 out]
      }
      event "Dual Screens": Value Change {
        n136 = event-data() -> ("NewVal"=w254:bool)  [unwired: 1 in, 5 out]
        n137 = property class="App"() -> ("Disp.AllMonitors"=w255:T12)  [unwired: 2 in, 2 out]
        n138 = control-ref of="This VI"() -> (w253:refnum<vi>)
        n139 = case shown="False" w254 {
          tunnel: w255 -> [w258 w271]
          tunnel: T8 {"Left"=0, "Top"=0, "Right"=0, "Bottom"=0} ("FP Window Bounds 2") -> [w257 w270]
          tunnel: w253 -> [_ w269]
          frame False {
            w261 = i16 0
            n140 = Index Array(array=w258, index=0) -> (element=w265:T13)
            n141 = Unbundle By Name(w265) -> ("Bounds.Right"=w266:i16, "Bounds.Bottom"=w263:i16, "Bounds.Top"=w262:i16)
            n142 = Subtract(x=w263, y=w262) -> (x-y=w260:i16)
            n143 = Bundle By Name(cluster=w257, "Left"=w261, "Top"=w261, "Right"=w266, "Bottom"=w260) -> (w259:T8)
            n144 = property class="VI"("Front Panel.WinBounds"=w259) -> (reference out=w268:refnum<vi>)  [unwired: 2 in, 1 out]
            n145 = property class="VI"(reference=w268, "FP.State"=T9."Maximized" ("Front Panel Window:State")) -> ()  [unwired: 1 in, 2 out]
          }
          frame True {
            w280 = i16 0
            n146 = Index Array(array=w271, index #1=1 ("index"), index #2=0 ("index")) -> (element #1=w274:T13, element #2=w275:T13)
            n147 = Unbundle By Name(w274) -> ("Bounds.Right"=w276:i16)
            n148 = Unbundle By Name(w275) -> ("Bounds.Left"=w277:i16, "Bounds.Bottom"=w278:i16, "Bounds.Top"=w279:i16)
            n149 = Subtract(x=w276, y=w277) -> (x-y=w281:i16)
            n150 = Subtract(x=w278, y=w279) -> (x-y=w282:i16)
            n151 = Bundle By Name(cluster=w270, "Left"=w280, "Top"=w280, "Right"=w281, "Bottom"=w282) -> (w283:T8)
            n152 = property class="VI"(reference=w269, "Front Panel.WinBounds"=w283) -> ()  [unwired: 1 in, 2 out]
          }
        }
      }
      event Value Change {
        n153 = event-data() -> ("OldVal"=w300:T4, "NewVal"=w284:T4)  [unwired: 1 in]
        n154 = Equal?(x=w300, y=w284) -> (x = y?=w301:bool)
        n155 = case shown="False" w301 {
          tunnel: w284 -> [w303 _]
          tunnel: w300 -> [w313 _]
          frame False {
            n156 = Unbundle By Name(w303) -> ("Image Format"=w314:u16, "Scan Mode"=w306:enum16{"XY", "XZ", "YZ", "XYZ"})
            n157 = Unbundle By Name(w313) -> ("Scan Mode"=w307:enum16{"XY", "XZ", "YZ", "XYZ"})
            n158 = call "Scan Parameters Action Engine.vi"("Action"=enum16{"Read", "Write"}."Read") -> ("Scan Parameters OUT"=w309:T5)  [unwired: 14 in]
            n159 = Bundle By Name(cluster=w309, "Last_Scan_Mode"=w307, "Current_Scan_Mode"=w306) -> (w304:T5)
            n160 = case shown="\"XY\", Default" w307 {
              tunnel: w314 -> [w319 w347 w375 w403]
              tunnel: w314 -> [w318 w346 w374 w402]
              tunnel: w306 -> [w320 w348 w376 w404]
              tunnel: [w317 w345 w373 w401] -> w312
              tunnel: [w316 w344 w372 w400] -> w311
              tunnel: [w315 w343 w371 w399] -> w310
              frame "XY", Default {
                n161 = case shown="\"XZ\"" w320 {
                  tunnel: w319 -> [w322 w329 w334 w336]
                  tunnel: w318 -> [w323 w326 w333 w340]
                  tunnel: [w322 w325 w331 w337] -> w317
                  tunnel: [w323 w324 w330 w341] -> w316
                  tunnel: [FALSE ("Cursor.Visible") TRUE ("Cursor.Visible") TRUE ("Cursor.Visible") FALSE ("Cursor.Visible")] -> w315
                  frame "XY", Default {
                  }
                  frame "XZ" {
                    n162 = Increment(x=w326) -> (x+1=w325:u16)
                    n163 = Divide(x=w329, y=2) -> (x/y=w324:dbl)
                  }
                  frame "YZ" {
                    n164 = Increment(x=w334) -> (x+1=w330:u16)
                    n165 = Divide(x=w333, y=2) -> (x/y=w331:dbl)
                  }
                  frame "XYZ" {
                    n166 = Divide(x=w340, y=2) -> (x/y=w341:dbl)
                    n167 = Divide(x=w336, y=2) -> (x/y=w337:dbl)
                  }
                }
              }
              frame "XZ" {
                n168 = case shown="\"XYZ\"" w348 {
                  tunnel: w347 -> [w350 w357 w361 w364]
                  tunnel: w346 -> [w352 w356 w359 w368]
                  tunnel: [w349 w357 w358 w365] -> w345
                  tunnel: [w351 w356 w360 w369] -> w344
                  tunnel: [TRUE ("Cursor.Visible") FALSE ("Cursor.Visible") TRUE ("Cursor.Visible") FALSE ("Cursor.Visible")] -> w343
                  frame "XY" {
                    n169 = Increment(x=w350) -> (x+1=w349:u16)
                    n170 = Divide(x=w352, y=2) -> (x/y=w351:dbl)
                  }
                  frame "XZ", Default {
                  }
                  frame "YZ" {
                    n171 = Increment(x=w359) -> (x+1=w360:u16)
                    n172 = Divide(x=w361, y=2) -> (x/y=w358:dbl)
                  }
                  frame "XYZ" {
                    n173 = Divide(x=w368, y=2) -> (x/y=w369:dbl)
                    n174 = Divide(x=w364, y=2) -> (x/y=w365:dbl)
                  }
                }
              }
              frame "YZ" {
                n175 = case shown="\"YZ\", Default" w376 {
                  tunnel: w375 -> [w378 w386 w389 w397]
                  tunnel: w374 -> [w380 w384 w393 w398]
                  tunnel: [w377 w383 w390 w397] -> w373
                  tunnel: [w379 w385 w394 w398] -> w372
                  tunnel: [TRUE ("Cursor.Visible") TRUE ("Cursor.Visible") FALSE ("Cursor.Visible") FALSE ("Cursor.Visible")] -> w371
                  frame "XY" {
                    n176 = Increment(x=w378) -> (x+1=w377:u16)
                    n177 = Divide(x=w380, y=2) -> (x/y=w379:dbl)
                  }
                  frame "XZ" {
                    n178 = Increment(x=w384) -> (x+1=w385:u16)
                    n179 = Divide(x=w386, y=2) -> (x/y=w383:dbl)
                  }
                  frame "XYZ" {
                    n180 = Divide(x=w393, y=2) -> (x/y=w394:dbl)
                    n181 = Divide(x=w389, y=2) -> (x/y=w390:dbl)
                  }
                  frame "YZ", Default {
                  }
                }
              }
              frame "XYZ" {
                n182 = case shown="\"XYZ\", Default" w404 {
                  tunnel: w403 -> [w405 w417 w422 w425]
                  tunnel: w402 -> [w409 w412 w419 w426]
                  tunnel: [w406 w416 w421 w425] -> w401
                  tunnel: [w410 w413 w420 w426] -> w400
                  tunnel: [FALSE ("Cursor.Visible") TRUE ("Cursor.Visible") TRUE ("Cursor.Visible") FALSE ("Cursor.Visible")] -> w399
                  frame "XY" {
                    n183 = Divide(x=w409, y=2) -> (x/y=w410:dbl)
                    n184 = Divide(x=w405, y=2) -> (x/y=w406:dbl)
                  }
                  frame "XZ" {
                    n185 = Increment(x=w412) -> (x+1=w413:u16)
                    n186 = Divide(x=w417, y=2) -> (x/y=w416:dbl)
                  }
                  frame "YZ" {
                    n187 = Increment(x=w422) -> (x+1=w421:u16)
                    n188 = Divide(x=w419, y=2) -> (x/y=w420:dbl)
                  }
                  frame "XYZ", Default {
                  }
                }
              }
            }
            n189 = property on="Channel 1" class="IntGraph (strict)"("Cursor.Cursor X"=w312, "Cursor.Cursor Y"=w311, "Cursor.Visible"=w310) -> ()  [unwired: 2 in, 2 out]
            n190 = call "Scan Parameters Action Engine.vi"("Action"=enum16{"Read", "Write"}."Write", "Scan Parameters IN"=w304) -> ()  [unwired: 13 in, 1 out]
          }
          frame True {
            n191 = property on="Channel 1" class="IntGraph (strict)"("Cursor.Visible"=FALSE) -> ()  [unwired: 2 in, 2 out]
          }
        }
        n192 = Unbundle By Name(w284) -> ("Image Dimension (um)"=w285:dbl[], "Scan Type"=w290:enum16{"Sample Scanning", "Beam Scanning"})
        n193 = Equal?(x=w290, y=enum16{"Sample Scanning", "Beam Scanning"}."Beam Scanning") -> (x = y?=w292:bool)
        n194 = Index Array(array=w285, index=0) -> (element=w293:dbl)
        n195 = call "Res Mirror um to Volts.vi"("Image Size (um)"=w293) -> ("Voltage (V)"=w294:dbl)
        n196 = In Range and Coerce(upper limit=4.8, x=w294, lower limit=0.0) -> (coerced(x)=w295:dbl)  [unwired: 1 out]
        n197 = call "Volts to I16.vi"("Voltage (V)"=w295) -> ("I16"=w289:i16)  [unwired: 13 in, 1 out]
        n198 = Bundle By Name(cluster=T3 {"Galvo 1 Position (I16)"=-280, "Galvo 2 Position (I16)"=-280, "X Axis Voltage (I16)"=0, "Y Axis Voltage (I16)"=0, "Z Axis Voltage (I16)"=0, "Res Mirror Amp (I16)"=0, "Res Mirror Mute"=FALSE} ("Manual Controls"), "Res Mirror Amp (I16)"=w289, "Res Mirror Mute"=w292) -> (w299:T3)
        n199 = call "FPGA-7842R-Control V1.vi"("Action"=FPGA-7842R-Reference."Set Res Mirror", "Manual Controls"=w299, "Initialize"=TRUE) -> ()  [unwired: 12 in, 1 out]
      }
      event "Unused Axis Voltage": Value Change {
        n200 = event-data() -> ()  [unwired: 1 in, 6 out]
        n201 = call "FPGA-7842R-Control V1.vi"("Action"=FPGA-7842R-Reference."Unused Axis I16", "Initialize"=TRUE, "Unused Axis Offset (I16)"="Unused Axis Voltage") -> ()  [unwired: 12 in, 1 out]
      }
      event "Set Mode Offset": Value Change {
        n202 = event-data() -> ("NewVal"=w432:bool)  [unwired: 1 in]
        n203 = case shown="True" w432 {
          frame False {
          }
          frame True {
            # "Vert Pixels"
            # "Horz Pixels"
            # "Z Pixel Size"
            # "XY Pixel Size"
            # "Z volts per um"
            # "XY volts per um"
            n204 = local read "Image Acquisition Parameters"() -> (w447:T4)
            n205 = Unbundle By Name(w447) -> ("Image Format"=w448:u16, "Image Dimension (um)"=w451:dbl[])
            n206 = call "Scanning Volts to Microns.vi"() -> ("Scanning Conversions OUT"=w436:T14)
            n207 = Unbundle By Name(w436) -> ("Stage X Axis (Volts/um)"=w435:dbl, "Stage Z Axis (Volts/um)"=w434:dbl)
            n208 = property on="Channel 1" class="IntGraph (strict)"() -> ("Cursor.Cursor X"=w442:dbl, "Cursor.Cursor Y"=w443:dbl)  [unwired: 2 in, 2 out]
            n209 = To Double Precision Float(number=w448) -> (double precision float=w439:dbl)
            n210 = call "Scan Parameters Action Engine.vi"("Action"=enum16{"Read", "Write"}."Read") -> ("Scan Parameters OUT"=w456:T5)  [unwired: 14 in]
            n211 = Divide(x=w451, y=w439) -> (x/y=w452:dbl[])
            n212 = Unbundle By Name(w456) -> ("Last_Scan_Mode"=w445:enum16{"XY", "XZ", "YZ", "XYZ"}, "Current_Scan_Mode"=w446:enum16{"XY", "XZ", "YZ", "XYZ"})
            n213 = Index Array(array=w452, index #1=0 ("index"), index #2=1 ("index")) -> (element #1=w453:dbl, element #2=w454:dbl)
            n214 = Divide(x=w439, y=2.0) -> (x/y=w438:dbl)
            n215 = case shown="\"XY\", Default" w445 {
              tunnel: w446 -> [w461 w524 w571 w618]
              tunnel: w442 -> [w462 w516 w563 w610]
              tunnel: w443 -> [w463 w517 w564 w611]
              tunnel: w438 -> [w469 w523 w570 w617]
              tunnel: w453 -> [w468 w522 w569 w616]
              tunnel: w434 -> [w466 w520 w567 w614]
              tunnel: w435 -> [w467 w521 w568 w615]
              tunnel: w454 -> [w465 w519 w566 w613]
              tunnel: w438 -> [w464 w518 w565 w612]
              tunnel: w456 -> [w460 w515 w562 w609]
              tunnel: [w459 w514 w561 w608] -> w457
              tunnel: [w458 w513 w560 w607] -> w441
              frame "XY", Default {
                # "XY Scan Mode"
                n216 = case shown="\"YZ\"" w461 {
                  tunnel: w469 -> [w478 _ w504 _]
                  tunnel: w468 -> [w480 w498 w509 _]
                  tunnel: w467 -> [w479 w496 w507 _]
                  tunnel: w466 -> [_ _ _ _]
                  tunnel: w465 -> [_ _ _ _]
                  tunnel: w464 -> [w476 w494 _ _]
                  tunnel: w463 -> [w477 w493 _ _]
                  tunnel: w462 -> [w485 _ w503 _]
                  tunnel: w460 -> [w484 w490 w502 w512]
                  tunnel: [w483 w491 w501 w512] -> w459
                  tunnel: [w488 w489 w500 w511] -> w458
                  frame "XY", Default {
                    # "XY - No change"
                    n217 = Unbundle By Name(w484) -> ("Stage_X_Off_V"=w474:dbl, "Stage_Y_Off_V"=w472:dbl, "Stage_Z_Off_V"=w488:dbl)
                    n218 = Subtract(x=w485, y=w478) -> (x-y=w487:dbl)
                    n219 = Multiply(x=w487, y=w480) -> (x*y=w486:dbl)
                    n220 = Multiply(x=w486, y=w479) -> (x*y=w475:dbl)
                    n221 = Subtract(x=w477, y=w476) -> (x-y=w481:dbl)
                    n222 = Multiply(x=w481, y=w480) -> (x*y=w482:dbl)
                    n223 = Add(x=w474, y=w475) -> (x+y=w473:dbl)
                    n224 = Multiply(x=w482, y=w479) -> (x*y=w471:dbl)
                    n225 = Add(x=w472, y=w471) -> (x+y=w470:dbl)
                    n226 = Bundle By Name(cluster=w484, "Stage_X_Off_V"=w473, "Stage_Y_Off_V"=w470) -> (w483:T5)
                  }
                  frame "XZ" {
                    # "XZ - Grab Y cusor position - Set Y offset"
                    n227 = Subtract(x=w493, y=w494) -> (x-y=w499:dbl)
                    n228 = Unbundle By Name(w490) -> ("Stage_Y_Off_V"=w492:dbl)
                    n229 = Multiply(x=w499, y=w498) -> (x*y=w497:dbl)
                    n230 = Multiply(x=w497, y=w496) -> (x*y=w495:dbl)
                    n231 = Add(x=w492, y=w495) -> (x+y=w489:dbl)
                    n232 = Bundle By Name(cluster=w490, "Stage_Y_Off_V"=w489) -> (w491:T5)
                  }
                  frame "YZ" {
                    # "YZ - Grab X cursor position - Set X offset"
                    n233 = Subtract(x=w503, y=w504) -> (x-y=w510:dbl)
                    n234 = Unbundle By Name(w502) -> ("Stage_X_Off_V"=w506:dbl)
                    n235 = Multiply(x=w510, y=w509) -> (x*y=w508:dbl)
                    n236 = Multiply(x=w508, y=w507) -> (x*y=w505:dbl)
                    n237 = Add(x=w506, y=w505) -> (x+y=w500:dbl)
                    n238 = Bundle By Name(cluster=w502, "Stage_X_Off_V"=w500) -> (w501:T5)
                  }
                  frame "XYZ" {
                    # "XYZ - No change"
                    n239 = Unbundle By Name(w512) -> ("Stage_Z_Off_V"=w511:dbl)
                  }
                }
              }
              frame "XZ" {
                # "XZ Scan Mode"
                n240 = case shown="\"YZ\"" w524 {
                  tunnel: w523 -> [_ _ w540 _]
                  tunnel: w522 -> [_ _ w547 _]
                  tunnel: w521 -> [_ _ w544 _]
                  tunnel: w520 -> [w527 _ _ w551]
                  tunnel: w515 -> [w534 w537 w546 w558]
                  tunnel: w519 -> [w526 _ _ w550]
                  tunnel: [w531 w537 w541 w555] -> w514
                  tunnel: w518 -> [w530 _ _ w554]
                  tunnel: w517 -> [w529 _ _ w553]
                  tunnel: w516 -> [_ _ w539 _]
                  tunnel: [w525 w536 w538 w549] -> w513
                  frame "XY", Default {
                    # "XY - Grab Y cusor position - Set Z offset"
                    n241 = Subtract(x=w529, y=w530) -> (x-y=w535:dbl)
                    n242 = Unbundle By Name(w534) -> ("Stage_Z_Off_V"=w528:dbl)
                    n243 = Multiply(x=w535, y=w526) -> (x*y=w533:dbl)
                    n244 = Multiply(x=w533, y=w527) -> (x*y=w532:dbl)
                    n245 = Add(x=w528, y=w532) -> (x+y=w525:dbl)
                    n246 = Bundle By Name(cluster=w534, "Stage_Z_Off_V"=w525) -> (w531:T5)
                  }
                  frame "XZ" {
                    # "XZ - No change"
                    n247 = Unbundle By Name(w537) -> ("Stage_Z_Off_V"=w536:dbl)
                  }
                  frame "YZ" {
                    # "YZ - Grab X cursor position - Set X offset"
                    n248 = Subtract(x=w539, y=w540) -> (x-y=w548:dbl)
                    n249 = Unbundle By Name(w546) -> ("Stage_X_Off_V"=w543:dbl)
                    n250 = Multiply(x=w548, y=w547) -> (x*y=w545:dbl)
                    n251 = Multiply(x=w545, y=w544) -> (x*y=w542:dbl)
                    n252 = Add(x=w543, y=w542) -> (x+y=w538:dbl)
                    n253 = Bundle By Name(cluster=w546, "Stage_X_Off_V"=w538) -> (w541:T5)
                  }
                  frame "XYZ" {
                    # "XYZ - Grab Y cusor position - Set Z offset"
                    n254 = Subtract(x=w553, y=w554) -> (x-y=w559:dbl)
                    n255 = Unbundle By Name(w558) -> ("Stage_Z_Off_V"=w552:dbl)
                    n256 = Multiply(x=w559, y=w550) -> (x*y=w557:dbl)
                    n257 = Multiply(x=w557, y=w551) -> (x*y=w556:dbl)
                    n258 = Add(x=w552, y=w556) -> (x+y=w549:dbl)
                    n259 = Bundle By Name(cluster=w558, "Stage_Z_Off_V"=w549) -> (w555:T5)
                  }
                }
              }
              frame "YZ" {
                # "YZ Scan Mode"
                n260 = case shown="\"XZ\"" w571 {
                  tunnel: w570 -> [_ w585 _ _]
                  tunnel: w569 -> [_ w592 _ _]
                  tunnel: w568 -> [_ w589 _ _]
                  tunnel: w567 -> [w574 _ _ w598]
                  tunnel: w562 -> [w581 w591 w595 w605]
                  tunnel: w566 -> [w573 _ _ w597]
                  tunnel: [w578 w586 w595 w602] -> w561
                  tunnel: w565 -> [w577 _ _ w601]
                  tunnel: w564 -> [w576 _ _ w600]
                  tunnel: w563 -> [_ w584 _ _]
                  tunnel: [w572 w583 w594 w596] -> w560
                  frame "XY", Default {
                    # "XY - Grab Y cusor position - Set Z offset"
                    n261 = Subtract(x=w576, y=w577) -> (x-y=w582:dbl)
                    n262 = Unbundle By Name(w581) -> ("Stage_Z_Off_V"=w575:dbl)
                    n263 = Multiply(x=w582, y=w573) -> (x*y=w580:dbl)
                    n264 = Multiply(x=w580, y=w574) -> (x*y=w579:dbl)
                    n265 = Add(x=w575, y=w579) -> (x+y=w572:dbl)
                    n266 = Bundle By Name(cluster=w581, "Stage_Z_Off_V"=w572) -> (w578:T5)
                  }
                  frame "XZ" {
                    # "XZ - Grab X cursor position - Set Y offset"
                    n267 = Subtract(x=w584, y=w585) -> (x-y=w593:dbl)
                    n268 = Unbundle By Name(w591) -> ("Stage_Y_Off_V"=w588:dbl)
                    n269 = Multiply(x=w593, y=w592) -> (x*y=w590:dbl)
                    n270 = Multiply(x=w590, y=w589) -> (x*y=w587:dbl)
                    n271 = Add(x=w588, y=w587) -> (x+y=w583:dbl)
                    n272 = Bundle By Name(cluster=w591, "Stage_Y_Off_V"=w583) -> (w586:T5)
                  }
                  frame "YZ" {
                    # "YZ - No change"
                    n273 = Unbundle By Name(w595) -> ("Stage_Z_Off_V"=w594:dbl)
                  }
                  frame "XYZ" {
                    # "XYZ - Grab Y cusor position - Set Z offset"
                    n274 = Subtract(x=w600, y=w601) -> (x-y=w606:dbl)
                    n275 = Unbundle By Name(w605) -> ("Stage_Z_Off_V"=w599:dbl)
                    n276 = Multiply(x=w606, y=w597) -> (x*y=w604:dbl)
                    n277 = Multiply(x=w604, y=w598) -> (x*y=w603:dbl)
                    n278 = Add(x=w599, y=w603) -> (x+y=w596:dbl)
                    n279 = Bundle By Name(cluster=w605, "Stage_Z_Off_V"=w596) -> (w602:T5)
                  }
                }
              }
              frame "XYZ" {
                # "XYZ Scan Mode"
                n280 = case shown="\"XZ\"" w618 {
                  tunnel: w617 -> [_ _ w634 _]
                  tunnel: w616 -> [_ w630 w641 _]
                  tunnel: w615 -> [_ w627 w638 _]
                  tunnel: w614 -> [_ _ _ _]
                  tunnel: w609 -> [w620 w629 w640 w644]
                  tunnel: w613 -> [_ _ _ _]
                  tunnel: [w620 w625 w635 w644] -> w608
                  tunnel: w612 -> [_ w624 _ _]
                  tunnel: w611 -> [_ w623 _ _]
                  tunnel: w610 -> [_ _ w633 _]
                  tunnel: [w619 w621 w632 w643] -> w607
                  frame "XY", Default {
                    # "XY - No change"
                    n281 = Unbundle By Name(w620) -> ("Stage_Z_Off_V"=w619:dbl)
                  }
                  frame "XZ" {
                    # "XZ - Grab Y cusor position - Set Y offset"
                    n282 = Subtract(x=w623, y=w624) -> (x-y=w631:dbl)
                    n283 = Unbundle By Name(w629) -> ("Stage_Y_Off_V"=w622:dbl)
                    n284 = Multiply(x=w631, y=w630) -> (x*y=w628:dbl)
                    n285 = Multiply(x=w628, y=w627) -> (x*y=w626:dbl)
                    n286 = Add(x=w622, y=w626) -> (x+y=w621:dbl)
                    n287 = Bundle By Name(cluster=w629, "Stage_Y_Off_V"=w621) -> (w625:T5)
                  }
                  frame "YZ" {
                    # "YZ - Grab X cursor position - Set X offset"
                    n288 = Subtract(x=w633, y=w634) -> (x-y=w642:dbl)
                    n289 = Unbundle By Name(w640) -> ("Stage_X_Off_V"=w637:dbl)
                    n290 = Multiply(x=w642, y=w641) -> (x*y=w639:dbl)
                    n291 = Multiply(x=w639, y=w638) -> (x*y=w636:dbl)
                    n292 = Add(x=w637, y=w636) -> (x+y=w632:dbl)
                    n293 = Bundle By Name(cluster=w640, "Stage_X_Off_V"=w632) -> (w635:T5)
                  }
                  frame "XYZ" {
                    # "XYZ - No change"
                    n294 = Unbundle By Name(w644) -> ("Stage_Z_Off_V"=w643:dbl)
                  }
                }
              }
            }
            n295 = call "Volts to I16.vi"("Voltage (V)"=w441) -> ("I16"=w440:i16)  [unwired: 13 in, 1 out]
            n296 = local write "Unused Axis Voltage"(w440) -> ()
            n297 = call "Scan Parameters Action Engine.vi"("Action"=enum16{"Read", "Write"}."Write", "Scan Parameters IN"=w457) -> ()  [unwired: 13 in, 1 out]
          }
        }
      }
      event "show cursor": Value Change {
        w646 = 50.0 ("Cursor.Cursor Position:Cursor X")
        n298 = event-data() -> ("NewVal"=w647:bool)  [unwired: 1 in, 5 out]
        n299 = property on="Channel 1" class="IntGraph (strict)"("Cursor.Cursor X"=w646, "Cursor.Cursor Y"=w646, "Cursor.Visible"=w647) -> ()  [unwired: 2 in, 2 out]
      }
    }
  }
  n300 = while {
    shift-right: [w656] -> _
    shift-left: "Idle" -> [w657]
    tunnel: w14 -> [w653]
    shift-right: [w651] -> _
    shift-left: w11 -> [w652]
    tunnel: w2 -> [w648]
    stop <- w655 stop-if-true
    n301 = case shown="\"Start Waveforms\"" w657 {
      selector: w657 -> [_ _ _ w687 _ _ _ _ _ _]
      tunnel: ["Exit" w664 "Idle" ("name (unnamed)") "Arange Displays" ("name (unnamed)") "Start FPGA Acquisition" ("name (unnamed)") "Display" ("name (unnamed)") "Close Images" ("name (unnamed)") "Idle" "Stop Waveforms" ("name (unnamed)") "Start Waveforms" ("name (unnamed)")] -> w656
      tunnel: [TRUE w666 w673 w695 w709 w721 w757 w790 w795 w801] -> w655
      tunnel: FALSE -> [_ w666 w673 w695 w709 w721 w757 w790 w795 w801]
      tunnel: w653 -> [_ w665 _ _ _ _ _ _ _ _]
      tunnel: w652 -> [w660 w663 w674 w693 w706 w719 w755 w788 w796 w802]
      tunnel: [w659 w663 w674 w693 w706 w714 w755 w787 w796 w802] -> w651
      tunnel: "Image Acquisition Parameters" -> [_ _ _ w686 _ w711 _ _ _ w799]
      tunnel: "Detectors" -> [_ _ _ w685 _ _ _ _ _ w797]
      tunnel: w648 -> [_ _ _ _ w702 _ _ _ _ _]
      frame "Exit" {
        n302 = call "FPGA-7842R-Control V1.vi"("Action"=FPGA-7842R-Reference."Close FPGA", "Initialize"=w660) -> ("Initalized"=w659:bool)  [unwired: 13 in]
      }
      frame "Idle", Default {
        n303 = Dequeue Element(queue=w665, timeout in ms (-1)=-1) -> (element=w664:string)  [unwired: 1 in, 3 out]
      }
      frame "Close Images" {
        w669 = u16 0 items=["Read", "Write"] ("Mode")
        w670 = u16 0 items=["Write", "Read"] ("Mode")
        n304 = call "File Action V1.vi"("Mode"=w669) -> ("Files Open"=w668:bool)  [unwired: 12 in, 2 out]
        n305 = call "Image_Actions_V1.vi"("Mode"=w670, "Action"="Trash Images") -> ()  [unwired: 12 in, 2 out]
        n306 = case shown="True" w668 {
          frame False {
          }
          frame True {
            w676 = u16 1 items=["Read", "Write"] ("Mode")
            n307 = call "File Action V1.vi"("Action"="Close Files", "Mode"=w676) -> ()  [unwired: 11 in, 3 out]
          }
        }
      }
      frame "Capture", "Live" {
        w691 = u16 0 items=["Write", "Read"] ("Mode")
        n308 = Cluster To Array(cluster=w685) -> (array=w683:bool[])
        n309 = Index Array(array=w683, index=4) -> (element=w680:bool)
        n310 = Boolean To (0,1)(Boolean=w683) -> (0, 1=w684:i16[])
        n311 = Add Array Elements(numeric array=w684) -> (sum=w681:i16)
        n312 = To Long Integer(number=w681) -> (32bit integer=w678:i32)
        n313 = Unbundle By Name(w686) -> ("Image Format"=w688:u16)
        n314 = Select(t=1, s=w680, f=w678) -> (s? t:f=w677:i32)
        n315 = case shown="Default" w687 {
          tunnel: w686 -> [_ w697]
          tunnel: w677 -> [_ w696]
          frame Default {
          }
          frame "Capture" {
            w700 = u16 1 items=["Read", "Write"] ("Mode")
            n316 = call "File Action V1.vi"("Action"="Open Files", "Mode"=w700, "Image Acquisition Parameters"=w697, "File Path IN"="Save File Path", "Number of Channels"=w696) -> ("File Path OUT"=w698:path)  [unwired: 8 in, 2 out]
            n317 = local write "Save File Path"(w698) -> ()
          }
        }
        n318 = To Long Integer(number=w688) -> (32bit integer=w690:i32)
        n319 = Bundle(w690, w690) -> (w689:cluster{i32, i32})  [unwired: 1 in]
        n320 = call "Image_Actions_V1.vi"("Image Size (Pixels)"=w689, "Mode"=w691, "Number of Channels"=w677, "Action"="Create Images") -> ()  [unwired: 10 in, 2 out]
      }
      frame "Arange Displays" {
        w704 = u16 1 items=["Write", "Read"] ("Mode")
        w708 = 1.0  # Aspect Ratio (h/w)
        w707 = u16 1 items=["Read", "Write"] ("Action")
        n321 = call "Image_Actions_V1.vi"("Mode"=w704) -> ("Image REFs OUT"=w705:T15[])  [unwired: 13 in, 1 out]
        n322 = Array Size(array=w705) -> (size(s)=w703:i32)
        n323 = call "Arange_Displays_V2.vi"("Display References"=w702, "Action"=w707, "Number of Channels"=w703, "Aspect Ratio (h/w)"=w708) -> ()  [unwired: 11 in, 1 out]
      }
      frame "Start Waveforms" {
        n324 = Unbundle By Name(w711) -> ("Scan Type"=w713:enum16{"Sample Scanning", "Beam Scanning"})
        n325 = case shown="\"Beam Scanning\"" w713 {
          tunnel: [w722 w723] -> w712
          frame "Sample Scanning", Default {
            n326 = local read "Unused Axis Voltage"() -> (w722:i16)
          }
          frame "Beam Scanning" {
            n327 = local read "Unused Axis Voltage"() -> (w723:i16)
          }
        }
        n328 = call "Initialize Waveforms V4.vi"("Image Acquisition Parameters"=w711) -> ("Waveform Data to FPGA"=w720:T16)  [unwired: 14 in]
        n329 = call "FPGA-7842R-Control V1.vi"("Waveform Data"=w720, "Action"=FPGA-7842R-Reference."Start Waveforms", "Image Acquisition Parameters"=w711, "Initialize"=w719) -> ("Initalized"=w715:bool)  [unwired: 11 in]
        n330 = call "FPGA-7842R-Control V1.vi"("Action"=FPGA-7842R-Reference."Unused Axis I16", "Initialize"=w715, "Unused Axis Offset (I16)"=w712) -> ("Initalized"=w714:bool)  [unwired: 12 in]
      }
      frame "Display" {
        w749 = u16 1 items=["Write", "Read"] ("Mode")
        n331 = call "Image_Actions_V1.vi"("Mode"=w749) -> ("Image REFs OUT"=w751:T15[])  [unwired: 13 in, 1 out]
        n332 = Array Size(array=w751) -> (size(s)=w747:i32)
        n333 = Decrement(x=w747) -> (x-1=w746:i32)
        n334 = for {
          N: 6 -> [_]
          tunnel: w746 -> [w785]
          tunnel: [w783] -> w750 mode=indexing
          i -> [w784]
          n335 = Greater Or Equal?(x=w785, y=w784) -> (x >= y?=w783:bool)
        }
        n336 = Obtain Notifier(name (unnamed)="Running", notification data type=FALSE) -> (notifier out=w754:refnum<notifier>)  [unwired: 2 in, 2 out]
        n337 = Index Array(array=w750, index #1=1 ("index"), index #2=2 ("index"), index #3=3 ("index"), index #4=4 ("index"), index #5=5 ("index")) -> (element #1=w735:bool, element #2=w734:bool, element #3=w733:bool, element #4=w732:bool, element #5=w731:bool)
        n338 = Index Array(array=w751, index #1=0 ("index"), index #2=1 ("index"), index #3=2 ("index"), index #4=3 ("index"), index #5=4 ("index"), index #6=5 ("index")) -> (element #1=w730:T15, element #2=w729:T15, element #3=w728:T15, element #4=w727:T15, element #5=w726:T15, element #6=w725:T15)
        n339 = while {
          tunnel: w735 -> [w772]
          tunnel: w734 -> [w771]
          tunnel: w733 -> [w767]
          tunnel: w732 -> [w764]
          tunnel: w731 -> [w763]
          tunnel: w730 -> [w770]
          tunnel: w729 -> [w769]
          tunnel: w728 -> [w768]
          tunnel: w727 -> [w766]
          tunnel: w726 -> [w760]
          tunnel: w725 -> [w765]
          tunnel: w754 -> [w762]
          stop <- w761 stop-if-true
          n340 = Get Notifier Status(notifier=w762) -> (current notification=w761:bool)  [unwired: 1 in, 4 out]
          n341 = case shown="False" w772 {
            tunnel: w769 -> [_ w782]
            frame False {
            }
            frame True {
              n342 = call "IMAQ ImageToArray"("Image"=w782) -> ("Image Pixels (Float)"=→"Channel 2":sgl[][])  [unwired: 3 in, 4 out]
            }
          }
          n343 = case shown="False" w771 {
            tunnel: w768 -> [_ w780]
            frame False {
            }
            frame True {
              n344 = call "IMAQ ImageToArray"("Image"=w780) -> ("Image Pixels (Float)"=→"Channel 3":sgl[][])  [unwired: 3 in, 4 out]
            }
          }
          n345 = call "IMAQ ImageToArray"("Image"=w770) -> ("Image Pixels (Float)"=→"Channel 1":sgl[][])  [unwired: 3 in, 4 out]
          n346 = Wait (ms)(milliseconds to wait=u32 30) -> ()  [unwired: 1 out]
          n347 = case shown="False" w767 {
            tunnel: w766 -> [_ w778]
            frame False {
            }
            frame True {
              n348 = call "IMAQ ImageToArray"("Image"=w778) -> ("Image Pixels (Float)"=→"Channel 4":sgl[][])  [unwired: 3 in, 4 out]
            }
          }
          n349 = case shown="False" w764 {
            tunnel: w760 -> [_ w776]
            frame False {
            }
            frame True {
              n350 = call "IMAQ ImageToArray"("Image"=w776) -> ("Image Pixels (Float)"=→"Channel 5":sgl[][])  [unwired: 3 in, 4 out]
            }
          }
          n351 = case shown="False" w763 {
            tunnel: w765 -> [_ w774]
            frame False {
            }
            frame True {
              n352 = call "IMAQ ImageToArray"("Image"=w774) -> ("Image Pixels (Float)"=→"Channel 6":sgl[][])  [unwired: 3 in, 4 out]
            }
          }
        }
      }
      frame "Stop Waveforms" {
        n353 = call "FPGA-7842R-Control V1.vi"("Action"=FPGA-7842R-Reference."Stop Waveforms", "Initialize"=w788) -> ("Initalized"=w787:bool)  [unwired: 13 in]
      }
      frame "Stop Acquisition" {
        n354 = call "FPGA-7842R-Control V1.vi"("Action"=FPGA-7842R-Reference."Laser Control", "Laser Controls"=T2 {"STED Power (V)"=0.0, "590 Power (V)"=0.0, "STED"=FALSE, "640 nm"=FALSE, "590 nm"=FALSE, "485 nm"=FALSE, "Manual Control"=FALSE} ("Laser Controls 2"), "Initialize"=TRUE) -> ()  [unwired: 12 in, 1 out]
      }
      frame "Start FPGA Acquisition" {
        n355 = Unbundle By Name(w799) -> ("Scan Type"=w798:enum16{"Sample Scanning", "Beam Scanning"})
        n356 = case shown="\"Sample Scanning\", Default" w798 {
          tunnel: w799 -> [w804 w812]
          tunnel: w797 -> [w803 w810]
          frame "Sample Scanning", Default {
            n357 = vi-ref "FPGA Sample Scanning V1.vi"() -> (w807:refnum<vi>)
            n358 = property class="VI Interface Type 0"(reference=w807) -> ("Path"=w805:path)  [unwired: 1 in, 2 out]
            n359 = Open VI Reference(type specifier VI Refnum (for type only)=w807, vi path=w805, options=128) -> (vi reference=w808:refnum<vi>)  [unwired: 3 in, 1 out]
            n360 = call-by-ref "Start Asynchronous Call"(reference=w808, "Detectors"=w803, "Image Acquisition Parameters"=w804) -> (reference out=w809:refnum<vi>)  [unwired: 2 in, 1 out]
            n361 = Close Reference(reference=w809) -> ()  [unwired: 1 in, 1 out]
          }
          frame "Beam Scanning" {
            n362 = vi-ref "FPGA Beam Scanning V1.vi"() -> (w815:refnum<vi>)
            n363 = property class="VI Interface Type 0"(reference=w815) -> ("Path"=w813:path)  [unwired: 1 in, 2 out]
            n364 = Open VI Reference(type specifier VI Refnum (for type only)=w815, vi path=w813, options=128) -> (vi reference=w811:refnum<vi>)  [unwired: 3 in, 1 out]
            n365 = call-by-ref "Start Asynchronous Call"(reference=w811, "Detectors"=w810, "Image Acquisition Parameters"=w812) -> (reference out=w816:refnum<vi>)  [unwired: 2 in, 1 out]
            n366 = Close Reference(reference=w816) -> ()  [unwired: 1 in, 1 out]
          }
        }
      }
    }
  }
